vi "AMC100 UI DLL.vi"() -> ()   [LabVIEW 2015]
panel:
  in  "stop":bool
  in  "deviceHandle":i32
  in  "Tab Control":enum32{"Navigation", "Interface", "About"}(tab)
  out "move out":bool caption="Move"
  in  "Positioner 2":u16(ring)=15 caption="Positioner" items=["ECGp5050", "ECGt5050", "ECR3030", "ECR4040", "ECR5050", "ECSx3030", "ECSx3040", "ECSx3050", "ECSx3060", "ECSx3070", "ECSx3080", "ECSx5050", "ECSxy5050", "ECSz3030", "ECSz5050", "EOP1", "EOP2"]
  out "in target range3":bool
  in  "Target Range 3":u32 caption="Target Range"
  in  "Reset Error 2":bool
  in  "Reset Error 3":bool
  out "Error 3":bool caption="Error"
  out "Error Message 3":string
  out "actor type 3":u16(ring) caption="Status" items=["linear positioner"=0, "goniometer"=1, "rotator"=2, "< error >"=9]
  out "actor type 2":u16(ring) caption="Status" items=["linear positioner"=0, "rotator"=1, "goniometer"=2, "< error >"=9]
  out "actor type":u16(ring) caption="Status" items=["linear positioner"=0, "rotator"=1, "goniometer"=2, "< error >"=9]
  out "EotLeftDetected3":bool caption="Status Eot BWD"
  out "EotrightDetected3":bool caption="Status Eot FWD"
  in  "EoT 3":bool=TRUE caption="Stop on EoT"
  out "EotLeftDetected2":bool caption="Status Eot BWD"
  out "EotrightDetected2":bool caption="Status Eot FWD"
  in  "EoT 2":bool=TRUE caption="Stop on EoT"
  in  "Move 3":bool
  out "MoveSignal 3":bool caption="Move"
  out "MoveSignal":bool caption="Move"
  out "ReferenceSignal":bool=TRUE
  in  "Axis 3":bool caption="Closed Loop Funktions"
  in  "Axis 2":bool caption="Closed Loop Funktions"
  in  "Target Position 3":i32 caption="Target Position [µm]"
  in  "Target Position 1":i32 caption="Target position [µm]"
  in  "Number of steps 3":i32=1 caption="Number of Steps"
  in  "Number of steps 2":i32=1 caption="Number of Steps"
  in  "Output 2":bool caption="Axis 2"
  in  "Move 2":bool
  in  "Move":bool
  out "ReferenceSignal 3":bool
  out "Reference 3":dbl caption="Reference position [µm]" format="%#_6f"
  in  "Output":bool=TRUE caption="Axis 1"
  out "Output Status 3":bool caption="Output Status"
  out "Error Message":string
  out "Error":bool
  in  "Output 3":bool caption="Axis 3"
  out "Output Status 1":bool=TRUE caption="Output Status"
  out "Position 3":dbl caption="Position [µm]" format="%#_10g"
  out "Output Status 2":bool caption="Output Status"
  in  "auto Reset 3":bool=TRUE caption="Auto Reset"
  in  "amplitude [V] 3":dbl=45.001 caption="Amplitude [V]" format="%#.3f"
  in  "frequency [Hz] 3":dbl=997.363 caption="Frequency [Hz]" format="%#.3f"
  out "Error 2":bool caption="Error"
  out "Error Message 2":string
  out "Connected 3":bool caption="Positioner Connected/Moving"
  in  "Single Step Left 3":bool caption="Open Loop Funktions"
  in  "Positioner 3":u16(ring)=15 caption="Positioner" items=["ECGp5050", "ECGt5050", "ECR3030", "ECR4040", "ECR5050", "ECSx3030", "ECSx3040", "ECSx3050", "ECSx3060", "ECSx3070", "ECSx3080", "ECSx5050", "ECSxy5050", "ECSz3030", "ECSz5050", "EOP1", "EOP2"]
  in  "Endless Left 3":bool caption="Continuous Backward"
  in  "Continuous Forward":bool
  in  "Single Step Right 3":bool caption="Step(s)"
  in  "Fixed DC 3":i32 caption="DC Level"
  out "move out 3":bool caption="Move"
  out "Position 2":i32 caption="Position [µm]"
  in  "amplitude [V] 2":dbl=45.001 caption="Amplitude [V]" format="%#.3f"
  in  "Reference Auto Update 3":bool=TRUE caption="Auto Update"
  in  "Amplitude [V]":dbl=45.001 format="%#.3f"
  in  "frequency [Hz] 2":dbl=997.363 caption="Frequency [Hz]" format="%#.3f"
  in  "Reference Auto Update 1":bool=TRUE caption="Auto Update"
  in  "Frequency [Hz]":dbl=1998.531 format="%#.3f"
  out "Connected 2":bool caption="Positioner Connected/Moving"
  in  "Single Step Left":bool caption="Open Loop Funktions"
  in  "Single Step Left 2":bool caption="Open Loop Funktions"
  in  "Single Step Right 2":bool caption="Step(s)"
  in  "Number of steps 1":i32=1 caption="Number of Steps"
  out "ReferenceSignal 2":bool
  in  "Single Step Right":bool caption="Step(s)"
  in  "Endless Left":bool caption="Continuous Backward"
  in  "Continuous Forward":bool
  in  "Endless Left 2":bool caption="Continuous Backward"
  out "EotLeftDetected1":bool caption="Status Eot BWD"
  out "EotrightDetected1":bool caption="Status Eot FWD"
  in  "EoT 1":bool caption="Stop on EoT"
  in  "Target position 2":i32 caption="Target Position [µm]"
  out "in target range2":bool
  in  "Continuous Forward":bool
  out "Reference 2":i32 caption="Reference position [µm]"
  in  "Fixed DC 2":i32 caption="DC Level"
  out "MoveSignal 2":bool caption="Move"
  out "in target range1":bool
  in  "Target Range 2":u32 caption="Target Range"
  in  "Target Range 1":u32 caption="Target Range"
  out "Reference":dbl=-7597148.0 caption="Reference position [µm]" format="%#_6f"
  out "Position":dbl=14701.126 caption="Position [µm]" format="%#_10f"
  in  "Axis 1":bool caption="Closed Loop Funktions"
  in  "auto Reset 1":bool=TRUE caption="Auto Reset"
  in  "Fixed DC 1":i32 caption="DC Level"
  out "move out 2":bool caption="Move"
  in  "auto Reset 2":bool=TRUE caption="Auto Reset"
  in  "Reference Auto Update 2":bool=TRUE caption="Auto Update"
  in  "Reset Error":bool
  in  "Axes halt":bool=TRUE
  out "Connected":bool=TRUE caption="Positioner Connected/Moving"
  in  "Positioner":u16(ring)=15 items=["ECGp5050", "ECGt5050", "ECR3030", "ECR4040", "ECR5050", "ECSx3030", "ECSx3040", "ECSx3050", "ECSx3060", "ECSx3070", "ECSx3080", "ECSx5050", "ECSxy5050", "ECSz3030", "ECSz5050", "EOP1", "EOP2"]
  in  "RT in move 3":bool=TRUE caption="Move"
  in  "Steps per pulse 3":i32 caption="Steps per pulse [Steps]"
  out "RT in move Signal 3":bool=TRUE caption="move"
  in  "Mode Input 3":u16(ring) caption="Mode" items=["Trigger (LVDS)"=11, "Trigger (LVTTL)"=10, "Stepper (LVDS)"=9, "Stepper (LVTTL)"=8, "AquadB (LVDS)"=1, "AquadB (LVTTL)"=0, "OFF"=15]
  in  "Loop Mode 3":u16(ring) caption="Loop mode" items=["closed-loop"=1, "open-loop"=0]
  in  "Change per pulse 3":i32 caption="Change per pulse  [u°/nm]"
  in  "RT in move 2":bool=TRUE caption="Move"
  in  "Steps per pulse 2":i32 caption="Steps per pulse [Steps]"
  out "RT in move Signal 2":bool=TRUE caption="move"
  in  "Mode Input 2":u16(ring) caption="Mode" items=["Trigger (LVDS)"=11, "Trigger (LVTTL)"=10, "Stepper (LVDS)"=9, "Stepper (LVTTL)"=8, "AquadB (LVDS)"=1, "AquadB (LVTTL)"=0, "OFF"=15]
  in  "Loop Mode 2":u16(ring) caption="Loop mode" items=["closed-loop"=1, "open-loop"=0]
  in  "Change per pulse 2":i32 caption="Change per pulse  [u°/nm]"
  in  "Output Mode":u16(ring) caption="Mode" items=["AquadB (LVTTL)", "AquadB (LVDS)"]
  in  "RT in move 1":bool=TRUE caption="Move"
  in  "AquadB Resolution 3":i32 caption="AquadB Resolution [nm]"
  in  "AqaudB clock 2":i32 caption="AquadB Clock [ns]"
  in  "AqaudB clock 1":i32 caption="AquadB Clock [ns]"
  in  "AquadB Resolution 2":i32 caption="AquadB Resolution [nm]"
  in  "AquadB out 1":bool caption="AquadB enable"
  in  "Steps per pulse 1":i32 caption="Steps per pulse [Steps]"
  in  "AquadB out 3":bool caption="AquadB enable"
  in  "AquadB in res 1":i32 caption="AquadB Resolution [nm]"
  in  "AquadB Resolution 1":i32 caption="AquadB Resolution [nm]"
  in  "AquadB out 2":bool caption="AquadB enable"
  in  "AqaudB clock 3":i32 caption="AquadB Clock [ns]"
  in  "Reset Error 6":bool
  in  "Reset Error 5":bool
  out "Error Message 5":string
  out "Error 5":bool caption="Error"
  out "Error Message 6":string
  out "Error 6":bool caption="Error"
  in  "AquadB in res 3":i32 caption="AquadB Resolution [nm]"
  in  "AquadB in res 2":i32 caption="AquadB Resolution [nm]"
  in  "Reset Error 4":bool
  out "RT in move Signal 1":bool=TRUE caption="move"
  in  "Mode Input 1":u16(ring) caption="Mode" items=["Trigger (LVDS)"=11, "Trigger (LVTTL)"=10, "Stepper (LVDS)"=9, "Stepper (LVTTL)"=8, "AquadB (LVDS)"=1, "AquadB (LVTTL)"=0, "OFF"=15]
  out "Error Message 4":string
  out "Error 4":bool caption="Error"
  in  "Loop Mode 1":u16(ring) caption="Loop mode" items=["closed-loop"=1, "open-loop"=0]
  in  "Change per pulse 1":i32 caption="Change per pulse [u°/nm]"
  in  "Reset Error 7":bool
  in  "Factory Reset":bool
  in  "Reboot":bool
  out "Error Message 7":string
  in  "Lock password":string
  in  "name":string="Test" caption="Device Name"
  in  "Access Password":string
  out "locked":bool
  out "authorized":bool
  out "Error 7":bool caption="Error"
  in  "Unlock":bool=TRUE
  out "Name":string caption="Device Name"
  out "Device type":string="AMC100/NUM"
  out "Mac Adress":string="70:B3:D5:D7:61:E1"
  out "Sn":string caption="Serial Number"
  out "ip":string="192.168.1.1" caption="IP Adress"
  out "Firmware":string caption="Firmware Version"
  out "FPGA":string caption="FPGA Version"
  # "Real Time Output"
  # "Real Time Input"
  # "Global Parameters"
  # "Axis 1"
  # "Axis 1"
  # "Axis 2"
  # "Axis 2"
  # "Axis 3"
  # "Axis 3"
  # "Device Info"
  # "Device Access"
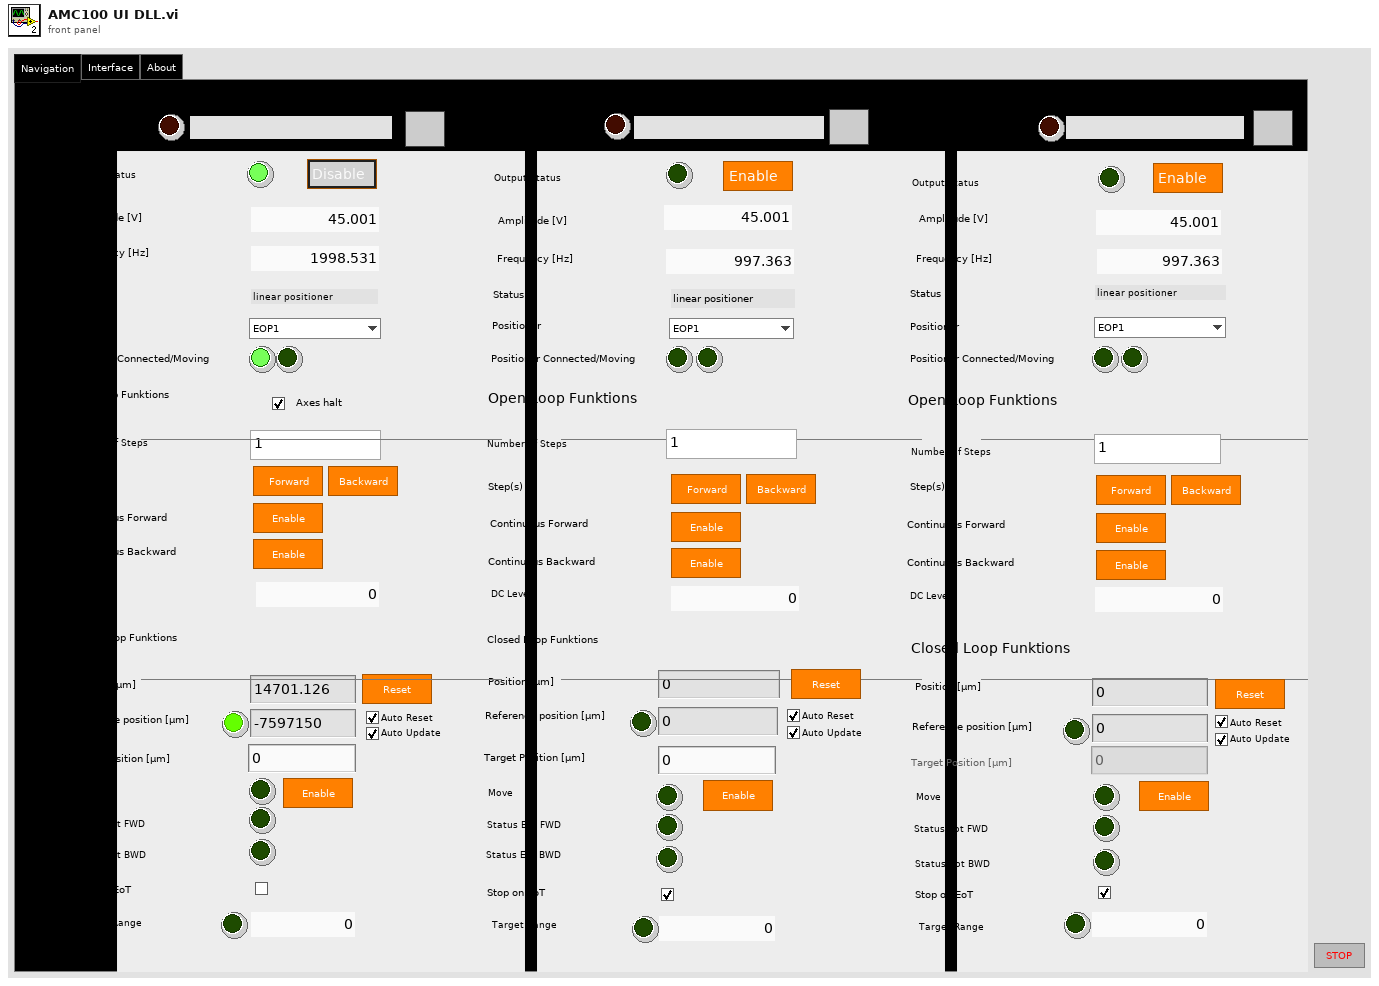
[diagram p1: front panel]
types:
  T1 = enum8{"Enabled", "Disabled", "Disabled and Grayed Out"}
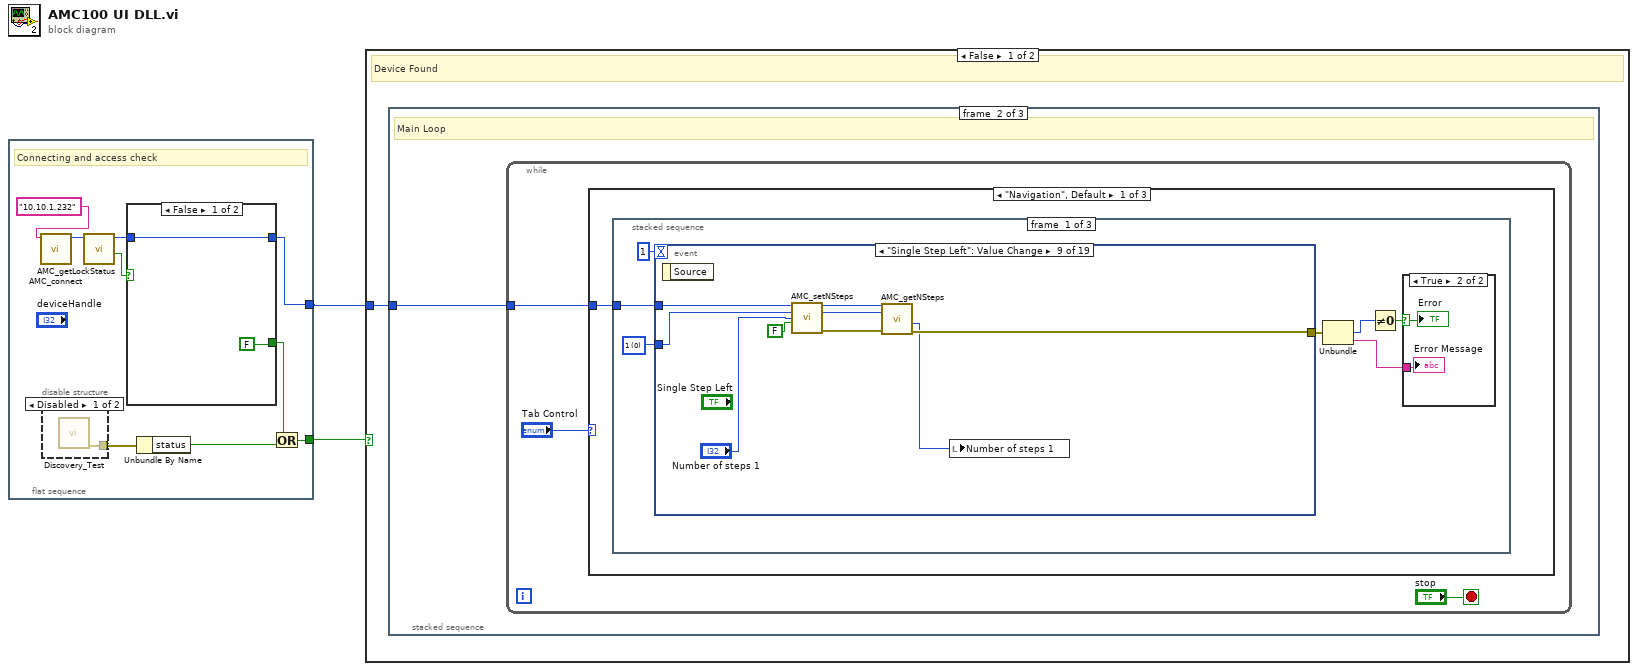
[diagram p0: block diagram]
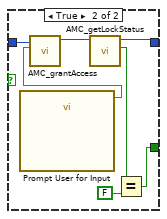
[diagram p3: hidden frame]
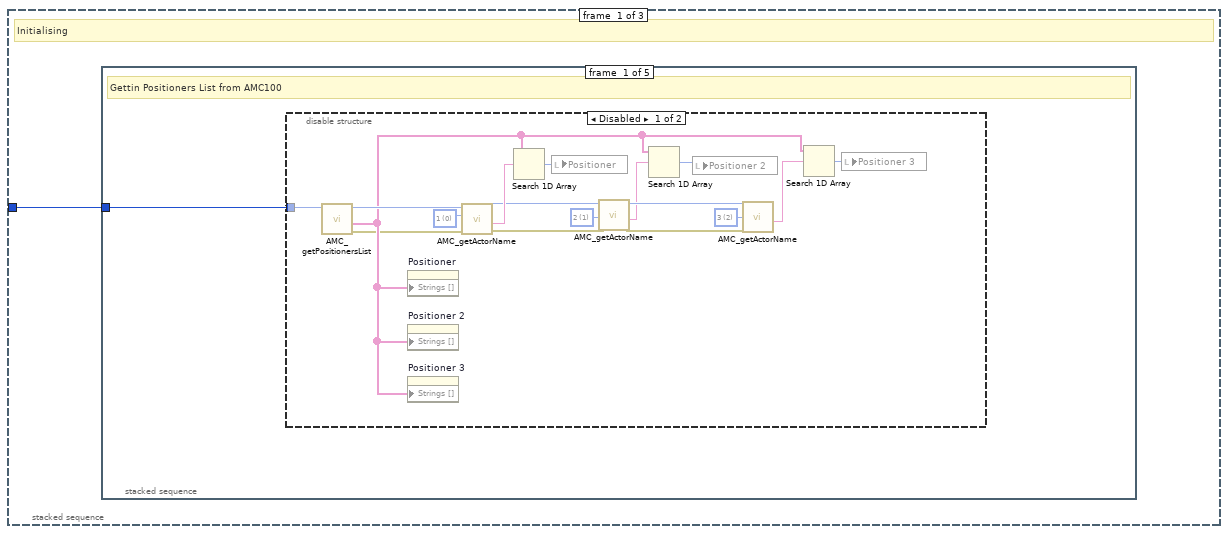
[diagram p4: hidden frame]
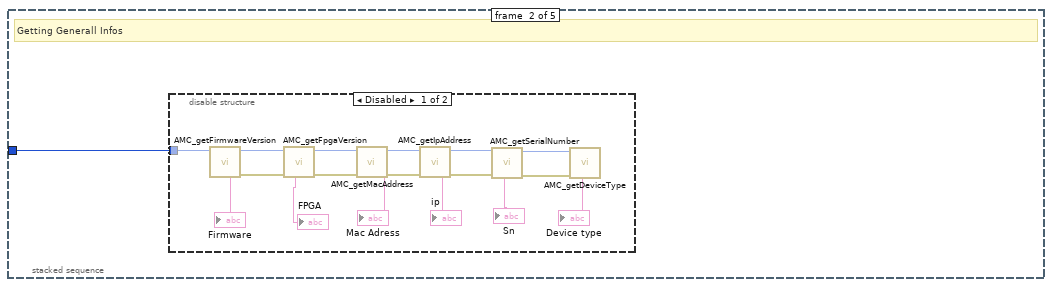
[diagram p6: hidden frame]
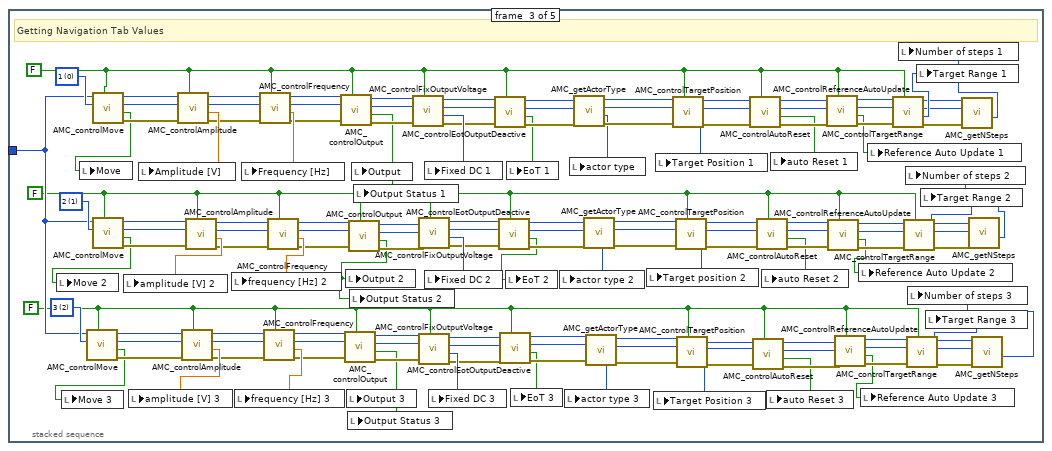
[diagram p8: hidden frame]
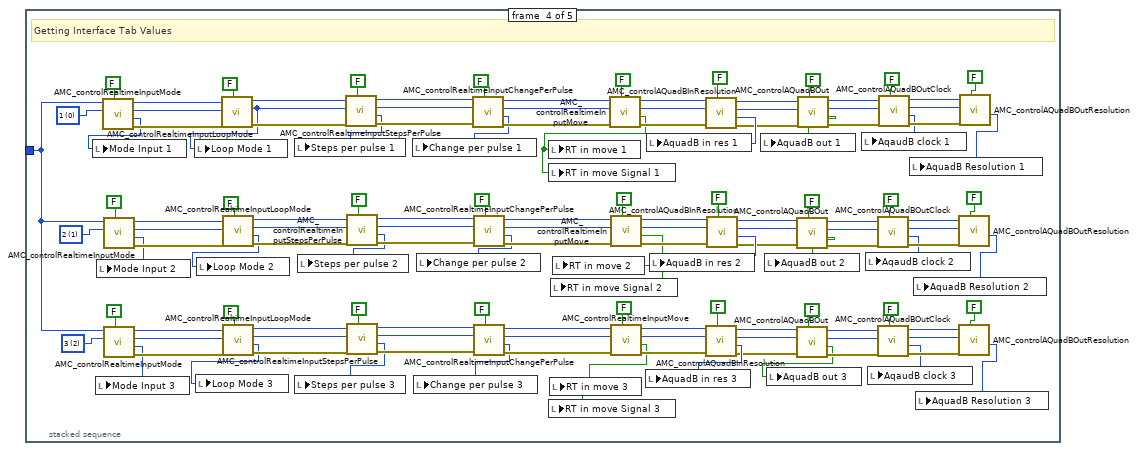
[diagram p9: hidden frame]
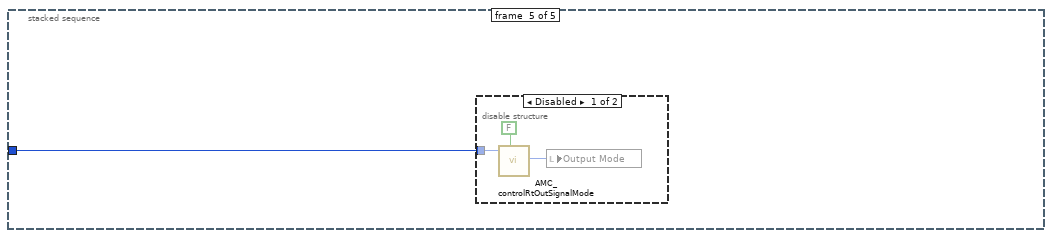
[diagram p10: hidden frame]
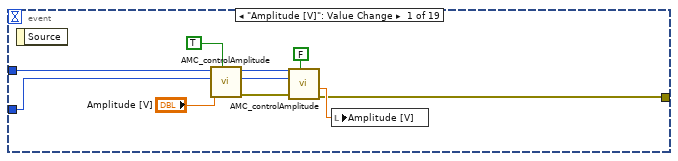
[diagram p13: hidden frame]
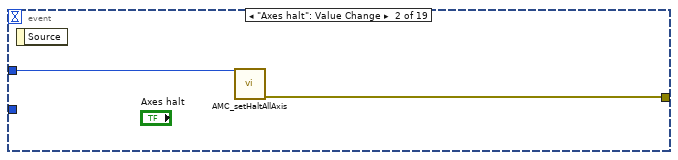
[diagram p14: hidden frame]
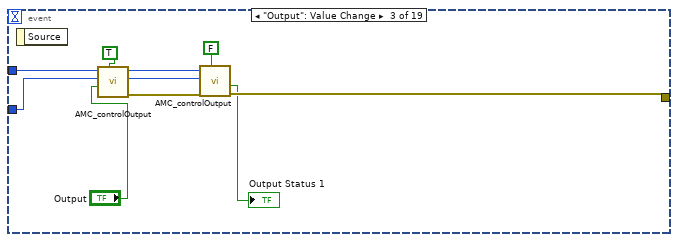
[diagram p15: hidden frame]
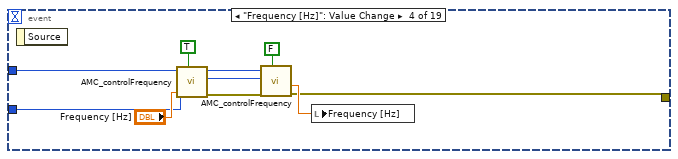
[diagram p16: hidden frame]
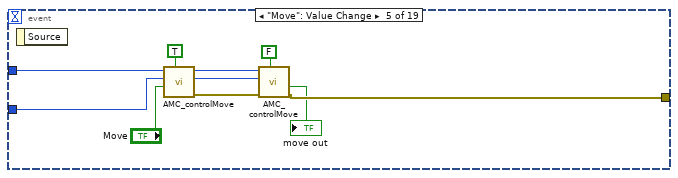
[diagram p17: hidden frame]
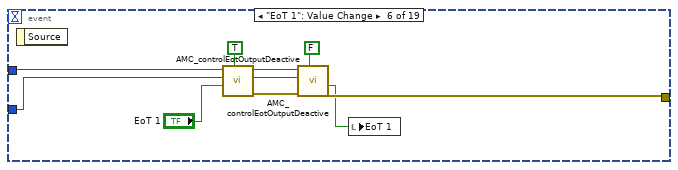
[diagram p18: hidden frame]
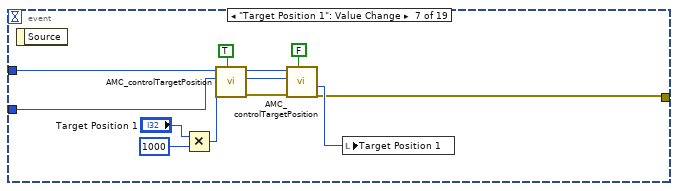
[diagram p19: hidden frame]
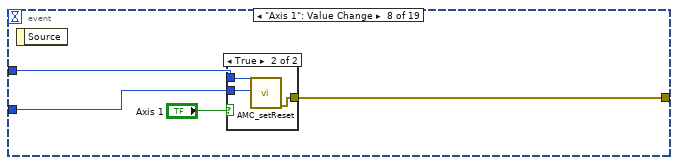
[diagram p20: hidden frame]
diagram:
  n1 = flat-sequence {
    tunnel: [w9] -> w1
    tunnel: [w10] -> w2
    frame #0 {
      # "Connecting and access check"
      n2 = call "AMC_connect.vi"("deviceAddress"="10.10.1.232") -> ("deviceHandle"=w6:i32)  [unwired: 5 in, 1 out]
      n3 = disable-structure shown="Disabled" {
        disable-tunnel: [w12 _] -> w11
        frame Disabled {
          n4 = call "Discovery_Test.vi"() -> ("error out"=w12:errorcluster)  [unwired: 10 in, 1 out]
        }
        frame Enabled {
        }
      }
      n5 = call "AMC_getLockStatus.vi"("deviceHandle"=w6) -> ("locked"=w4:bool, "deviceHandle"=w5:i32)  [unwired: 7 in, 2 out]
      n6 = case shown="False" w4 {
        tunnel: w5 -> [w14 w21]
        tunnel: [w14 w18] -> w10
        tunnel: [FALSE w15] -> w8
        frame False {
        }
        frame True {
          n7 = call "Prompt User for Input"() -> ("password"=w20:string)  [unwired: 17 in, 2 out]
          n8 = call "AMC_grantAccess.vi"("password"=w20, "deviceHandle"=w21) -> ("deviceHandle"=w19:i32)  [unwired: 8 in, 1 out]
          n9 = call "AMC_getLockStatus.vi"("deviceHandle"=w19) -> ("authorized"=w16:bool, "deviceHandle"=w18:i32)  [unwired: 7 in, 2 out]
          n10 = Equal?(x=w16, y=FALSE) -> (x = y?=w15:bool)
        }
      }
      n11 = Unbundle By Name(w11) -> ("status"=w7:bool)
      n12 = Or(x=w8, y=w7) -> (x .or. y?=w9:bool)
    }
  }
  n13 = case shown="False" w1 {
    tunnel: w2 -> [w22 _]
    frame False {
      # "Device Found"
      n14 = stacked-sequence {
        tunnel: w22 -> [w23 w335 w1339]
        frame #0 {
          # "Initialising"
          n15 = stacked-sequence {
            tunnel: w23 -> [w24 w42 w105 w281 w331]
            frame #0 {
              # "Gettin Positioners List from AMC100"
              n16 = disable-structure shown="Disabled" {
                disable-tunnel: w24 -> [w34 _]
                frame Disabled {
                  w36 = u8 2 items=["1", "2", "3"] ("axis")
                  w35 = u8 1 items=["1", "2", "3"] ("axis")
                  w39 = u8 0 items=["1", "2", "3"] ("axis")
                  n17 = call "AMC_getPositionersList.vi"("deviceHandle"=w34) -> ("error out"=w25:errorcluster, "list"=w28:string[], "deviceHandle"=w29:i32)  [unwired: 7 in, 1 out]
                  n18 = property on="Positioner" class="Ring (strict)"("Strings []"=w28) -> ()  [unwired: 2 in, 2 out]
                  n19 = property on="Positioner 2" class="Ring (strict)"("Strings []"=w28) -> ()  [unwired: 2 in, 2 out]
                  n20 = property on="Positioner 3" class="Ring (strict)"("Strings []"=w28) -> ()  [unwired: 2 in, 2 out]
                  n21 = call "AMC_getActorName.vi"("error in"=w25, "axis"=w39, "deviceHandle"=w29) -> ("error out"=w27:errorcluster, "actor name"=w40:string, "deviceHandle"=w38:i32)  [unwired: 5 in, 1 out]
                  n22 = Search 1D Array(1D array=w28, element=w40) -> (index of element=w41:i32)  [unwired: 1 in]
                  n23 = local write "Positioner"(w41) -> ()
                  n24 = call "AMC_getActorName.vi"("error in"=w27, "axis"=w35, "deviceHandle"=w38) -> ("error out"=w26:errorcluster, "actor name"=w31:string, "deviceHandle"=w37:i32)  [unwired: 5 in, 1 out]
                  n25 = Search 1D Array(1D array=w28, element=w31) -> (index of element=w33:i32)  [unwired: 1 in]
                  n26 = local write "Positioner 2"(w33) -> ()
                  n27 = call "AMC_getActorName.vi"("error in"=w26, "axis"=w36, "deviceHandle"=w37) -> ("actor name"=w30:string)  [unwired: 5 in, 3 out]
                  n28 = Search 1D Array(1D array=w28, element=w30) -> (index of element=w32:i32)  [unwired: 1 in]
                  n29 = local write "Positioner 3"(w32) -> ()
                }
                frame Enabled {
                }
              }
            }
            frame #1 {
              # "Getting Generall Infos"
              n30 = disable-structure shown="Disabled" {
                disable-tunnel: w42 -> [w47 _]
                frame Disabled {
                  n31 = call "AMC_getFirmwareVersion.vi"("deviceHandle"=w47) -> ("error out"=w45:errorcluster, "version"=→"Firmware":string, "deviceHandle"=w46:i32)  [unwired: 8 in]
                  n32 = call "AMC_getFpgaVersion.vi"("error in"=w45, "device Handle"=w46) -> ("error out"=w55:errorcluster, "version"=→"FPGA":string, "device Handle"=w59:i32)  [unwired: 7 in]
                  n33 = call "AMC_getMacAddress.vi"("error in"=w55, "deviceHandle"=w59) -> ("error out"=w54:errorcluster, "mac"=→"Mac Adress":string, "deviceHandle"=w57:i32)  [unwired: 7 in]
                  n34 = call "AMC_getIpAddress.vi"("error in"=w54, "device Handle"=w57) -> ("error out"=w51:errorcluster, "ip"=→"ip":string, "device Handle"=w52:i32)  [unwired: 7 in]
                  n35 = call "AMC_getSerialNumber.vi"("error in"=w51, "device Handle"=w52) -> ("error out"=w48:errorcluster, "sn"=→"Sn":string, "device Handle"=w49:i32)  [unwired: 7 in]
                  n36 = call "AMC_getDeviceType.vi"("error in"=w48, "device Handle"=w49) -> ("type"=→"Device type":string)  [unwired: 7 in, 2 out]
                }
                frame Enabled {
                }
              }
            }
            frame #2 {
              w106 = u8 2 items=["1", "2", "3"] ("axis")
              w93 = FALSE ("set")
              w107 = u8 1 items=["1", "2", "3"] ("axis")
              w94 = FALSE ("set")
              w108 = u8 0 items=["1", "2", "3"] ("axis")
              w95 = FALSE ("set")
              # "Getting Navigation Tab Values"
              n37 = call "AMC_controlMove.vi"("set"=w93, "axis"=w106, "deviceHandle"=w105) -> ("error out"=w109:errorcluster, "enable out"=w76:bool, "axis"=w110:u8, "deviceHandle"=w111:i32)  [unwired: 5 in]
              n38 = local write "Move 3"(w76) -> ()
              n39 = call "AMC_controlMove.vi"("set"=w95, "axis"=w108, "deviceHandle"=w105) -> ("error out"=w117:errorcluster, "enable out"=w86:bool, "axis"=w115:u8, "deviceHandle"=w116:i32)  [unwired: 5 in]
              n40 = local write "Move"(w86) -> ()
              n41 = call "AMC_controlMove.vi"("set"=w94, "axis"=w107, "deviceHandle"=w105) -> ("error out"=w112:errorcluster, "enable out"=w81:bool, "axis"=w113:u8, "deviceHandle"=w114:i32)  [unwired: 5 in]
              n42 = local write "Move 2"(w81) -> ()
              n43 = call "AMC_controlAmplitude.vi"("set"=w95, "error in"=w117, "axis"=w115, "deviceHandle"=w116) -> ("error out"=w174:errorcluster, "amplitude [V] out"=w200:dbl, "axis"=w186:u8, "deviceHandle"=w201:i32)  [unwired: 2 in]
              n44 = local write "Amplitude [V]"(w200) -> ()
              n45 = call "AMC_controlAmplitude.vi"("set"=w93, "error in"=w109, "axis"=w110, "deviceHandle"=w111) -> ("error out"=w168:errorcluster, "amplitude [V] out"=w191:dbl, "axis"=w180:u8, "deviceHandle"=w195:i32)  [unwired: 2 in]
              n46 = local write "amplitude [V] 3"(w191) -> ()
              n47 = call "AMC_controlAmplitude.vi"("set"=w94, "error in"=w112, "axis"=w113, "deviceHandle"=w114) -> ("error out"=w171:errorcluster, "amplitude [V] out"=w193:dbl, "axis"=w183:u8, "deviceHandle"=w197:i32)  [unwired: 2 in]
              n48 = local write "amplitude [V] 2"(w193) -> ()
              n49 = call "AMC_controlFrequency.vi"("set"=w95, "error in"=w174, "axis"=w186, "deviceHandle"=w201) -> ("error out"=w173:errorcluster, "frequency [Hz] out"=w199:dbl, "axis"=w185:u8, "deviceHandle"=w198:i32)  [unwired: 4 in]
              n50 = local write "Frequency [Hz]"(w199) -> ()
              n51 = call "AMC_controlFrequency.vi"("set"=w93, "error in"=w168, "axis"=w180, "deviceHandle"=w195) -> ("error out"=w167:errorcluster, "frequency [Hz] out"=w190:dbl, "axis"=w179:u8, "deviceHandle"=w194:i32)  [unwired: 4 in]
              n52 = local write "frequency [Hz] 3"(w190) -> ()
              n53 = call "AMC_controlFrequency.vi"("set"=w94, "error in"=w171, "axis"=w183, "deviceHandle"=w197) -> ("error out"=w170:errorcluster, "frequency [Hz] out"=w192:dbl, "axis"=w182:u8, "deviceHandle"=w196:i32)  [unwired: 4 in]
              n54 = local write "frequency [Hz] 2"(w192) -> ()
              n55 = call "AMC_controlOutput.vi"("set"=w95, "error in"=w173, "axis"=w185, "deviceHandle"=w198) -> ("error out"=w172:errorcluster, "enable out"=w85:bool, "axis"=w184:u8, "deviceHandle"=w189:i32)  [unwired: 4 in]
              n56 = call "AMC_controlOutput.vi"("set"=w93, "error in"=w167, "axis"=w179, "deviceHandle"=w194) -> ("error out"=w166:errorcluster, "enable out"=w75:bool, "axis"=w178:u8, "deviceHandle"=w187:i32)  [unwired: 4 in]
              n57 = local write "Output 3"(w75) -> ()
              n58 = local write "Output Status 3"(w75) -> ()
              n59 = call "AMC_controlOutput.vi"("set"=w94, "error in"=w170, "axis"=w182, "deviceHandle"=w196) -> ("error out"=w169:errorcluster, "enable out"=w80:bool, "axis"=w181:u8, "deviceHandle"=w188:i32)  [unwired: 4 in]
              n60 = local write "Output 2"(w80) -> ()
              n61 = local write "Output Status 2"(w80) -> ()
              n62 = local write "Output"(w85) -> ()
              n63 = local write "Output Status 1"(w85) -> ()
              n64 = call "AMC_controlFixOutputVoltage.vi"("set"=w95, "error in"=w172, "axis"=w184, "deviceHandle"=w189) -> ("error out"=w163:errorcluster, "voltage"=w177:i32, "axis"=w164:u8, "deviceHandle"=w165:i32)  [unwired: 4 in]
              n65 = call "AMC_controlFixOutputVoltage.vi"("set"=w94, "error in"=w169, "axis"=w181, "deviceHandle"=w188) -> ("error out"=w160:errorcluster, "voltage"=w176:i32, "axis"=w161:u8, "deviceHandle"=w162:i32)  [unwired: 4 in]
              n66 = call "AMC_controlFixOutputVoltage.vi"("set"=w93, "error in"=w166, "axis"=w178, "deviceHandle"=w187) -> ("error out"=w157:errorcluster, "voltage"=w175:i32, "axis"=w158:u8, "deviceHandle"=w159:i32)  [unwired: 4 in]
              n67 = local write "Fixed DC 1"(w177) -> ()
              n68 = local write "Fixed DC 2"(w176) -> ()
              n69 = local write "Fixed DC 3"(w175) -> ()
              n70 = call "AMC_controlEotOutputDeactive.vi"("set"=w95, "error in"=w163, "axis"=w164, "deviceHandle"=w165) -> ("error out"=w154:errorcluster, "enable out"=w84:bool, "axis"=w155:u8, "deviceHandle"=w156:i32)  [unwired: 4 in]
              n71 = call "AMC_controlEotOutputDeactive.vi"("set"=w94, "error in"=w160, "axis"=w161, "deviceHandle"=w162) -> ("error out"=w151:errorcluster, "enable out"=w79:bool, "axis"=w152:u8, "deviceHandle"=w153:i32)  [unwired: 4 in]
              n72 = call "AMC_controlEotOutputDeactive.vi"("set"=w93, "error in"=w157, "axis"=w158, "deviceHandle"=w159) -> ("error out"=w148:errorcluster, "enable out"=w74:bool, "axis"=w149:u8, "deviceHandle"=w150:i32)  [unwired: 4 in]
              n73 = local write "EoT 2"(w79) -> ()
              n74 = local write "EoT 1"(w84) -> ()
              n75 = local write "EoT 3"(w74) -> ()
              n76 = call "AMC_getActorType.vi"("error in"=w154, "axis"=w155, "deviceHandle"=w156) -> ("error out"=w142:errorcluster, "positioner type"=w89:u16, "axis"=w143:i32, "deviceHandle"=w144:i32)  [unwired: 5 in]
              n77 = local write "actor type"(w89) -> ()
              n78 = call "AMC_getActorType.vi"("error in"=w151, "axis"=w152, "deviceHandle"=w153) -> ("error out"=w145:errorcluster, "positioner type"=w88:u16, "axis"=w146:i32, "deviceHandle"=w147:i32)  [unwired: 5 in]
              n79 = local write "actor type 2"(w88) -> ()
              n80 = call "AMC_getActorType.vi"("error in"=w148, "axis"=w149, "deviceHandle"=w150) -> ("error out"=w139:errorcluster, "positioner type"=w87:u16, "axis"=w140:i32, "deviceHandle"=w141:i32)  [unwired: 5 in]
              n81 = local write "actor type 3"(w87) -> ()
              n82 = call "AMC_controlTargetPosition.vi"("set"=w95, "error in"=w142, "axis"=w143, "deviceHandle"=w144) -> ("error out"=w135:errorcluster, "target out"=w138:i32, "axis"=w131:u8, "deviceHandle"=w133:i32)  [unwired: 4 in]
              n83 = local write "Target Position 1"(w138) -> ()
              n84 = call "AMC_controlTargetPosition.vi"("set"=w94, "error in"=w145, "axis"=w146, "deviceHandle"=w147) -> ("error out"=w129:errorcluster, "target out"=w137:i32, "axis"=w125:u8, "deviceHandle"=w127:i32)  [unwired: 4 in]
              n85 = local write "Target position 2"(w137) -> ()
              n86 = call "AMC_controlTargetPosition.vi"("set"=w93, "error in"=w139, "axis"=w140, "deviceHandle"=w141) -> ("error out"=w123:errorcluster, "target out"=w136:i32, "axis"=w119:u8, "deviceHandle"=w121:i32)  [unwired: 4 in]
              n87 = local write "Target Position 3"(w136) -> ()
              n88 = call "AMC_controlAutoReset.vi"("set"=w95, "error in"=w135, "axis"=w131, "deviceHandle in"=w133) -> ("error out"=w134:errorcluster, "enable out"=w83:bool, "axis"=w130:u8, "deviceHandle out"=w132:i32)  [unwired: 4 in]
              n89 = call "AMC_controlAutoReset.vi"("set"=w93, "error in"=w123, "axis"=w119, "deviceHandle in"=w121) -> ("error out"=w122:errorcluster, "enable out"=w73:bool, "axis"=w118:u8, "deviceHandle out"=w120:i32)  [unwired: 4 in]
              n90 = call "AMC_controlAutoReset.vi"("set"=w94, "error in"=w129, "axis"=w125, "deviceHandle in"=w127) -> ("error out"=w128:errorcluster, "enable out"=w78:bool, "axis"=w124:u8, "deviceHandle out"=w126:i32)  [unwired: 4 in]
              n91 = local write "auto Reset 2"(w78) -> ()
              n92 = local write "auto Reset 3"(w73) -> ()
              n93 = local write "auto Reset 1"(w83) -> ()
              n94 = call "AMC_controlReferenceAutoUpdate.vi"("set"=w95, "error in"=w134, "axis"=w130, "deviceHandle"=w132) -> ("error out"=w102:errorcluster, "enable out"=w82:bool, "axis"=w103:u8, "deviceHandle"=w104:i32)  [unwired: 4 in]
              n95 = call "AMC_controlReferenceAutoUpdate.vi"("set"=w94, "error in"=w128, "axis"=w124, "deviceHandle"=w126) -> ("error out"=w99:errorcluster, "enable out"=w77:bool, "axis"=w100:u8, "deviceHandle"=w101:i32)  [unwired: 4 in]
              n96 = call "AMC_controlReferenceAutoUpdate.vi"("set"=w93, "error in"=w122, "axis"=w118, "deviceHandle"=w120) -> ("error out"=w96:errorcluster, "enable out"=w72:bool, "axis"=w97:u8, "deviceHandle"=w98:i32)  [unwired: 4 in]
              n97 = local write "Reference Auto Update 2"(w77) -> ()
              n98 = local write "Reference Auto Update 3"(w72) -> ()
              n99 = local write "Reference Auto Update 1"(w82) -> ()
              n100 = call "AMC_controlTargetRange.vi"("set"=w95, "error in"=w102, "axis"=w103, "deviceHandle"=w104) -> ("error out"=w69:errorcluster, "range out"=w92:u32, "axis"=w70:u8, "deviceHandle"=w71:i32)  [unwired: 4 in]
              n101 = call "AMC_controlTargetRange.vi"("set"=w94, "error in"=w99, "axis"=w100, "deviceHandle"=w101) -> ("error out"=w61:errorcluster, "range out"=w91:u32, "axis"=w67:u8, "deviceHandle"=w68:i32)  [unwired: 4 in]
              n102 = call "AMC_controlTargetRange.vi"("set"=w93, "error in"=w96, "axis"=w97, "deviceHandle"=w98) -> ("error out"=w60:errorcluster, "range out"=w90:u32, "axis"=w65:u8, "deviceHandle"=w66:i32)  [unwired: 4 in]
              n103 = local write "Target Range 1"(w92) -> ()
              n104 = local write "Target Range 2"(w91) -> ()
              n105 = local write "Target Range 3"(w90) -> ()
              n106 = call "AMC_getNSteps.vi"("error in"=w69, "axis"=w70, "deviceHandle"=w71) -> ("n out"=w63:i32)  [unwired: 5 in, 3 out]
              n107 = local write "Number of steps 1"(w63) -> ()
              n108 = call "AMC_getNSteps.vi"("error in"=w61, "axis"=w67, "deviceHandle"=w68) -> ("n out"=w64:i32)  [unwired: 5 in, 3 out]
              n109 = local write "Number of steps 2"(w64) -> ()
              n110 = call "AMC_getNSteps.vi"("error in"=w60, "axis"=w65, "deviceHandle"=w66) -> ("n out"=w62:i32)  [unwired: 5 in, 3 out]
              n111 = local write "Number of steps 3"(w62) -> ()
            }
            frame #3 {
              w279 = u8 2 items=["1", "2", "3"] ("axis")
              w280 = u8 1 items=["1", "2", "3"] ("axis")
              w314 = u8 0 items=["1", "2", "3"] ("axis")
              # "Getting Interface Tab Values"
              n112 = call "AMC_controlRealtimeInputMode.vi"("set"=FALSE, "axis"=w314, "deviceHandle"=w281) -> ("error out"=w319:errorcluster, "mode out"=w264:i32, "axis"=w278:u8, "deviceHandle"=w324:i32)  [unwired: 5 in]
              n113 = local write "Mode Input 1"(w264) -> ()
              n114 = call "AMC_controlRealtimeInputMode.vi"("set"=FALSE, "axis"=w280, "deviceHandle"=w281) -> ("error out"=w309:errorcluster, "mode out"=w258:i32, "axis"=w274:u8, "deviceHandle"=w304:i32)  [unwired: 5 in]
              n115 = local write "Mode Input 2"(w258) -> ()
              n116 = call "AMC_controlRealtimeInputMode.vi"("set"=FALSE, "axis"=w279, "deviceHandle"=w281) -> ("error out"=w286:errorcluster, "mode out"=w252:i32, "axis"=w269:u8, "deviceHandle"=w291:i32)  [unwired: 5 in]
              n117 = local write "Mode Input 3"(w252) -> ()
              n118 = call "AMC_controlRealtimeInputLoopMode.vi"("set"=FALSE, "error in"=w319, "axis"=w278, "deviceHandle"=w324) -> ("error out"=w318:errorcluster, "axis"=w263:u8, "deviceHandle"=w323:i32)  [unwired: 4 in, 1 out]
              n119 = local write "Loop Mode 1"(w263) -> ()
              n120 = call "AMC_controlRealtimeInputLoopMode.vi"("set"=FALSE, "error in"=w309, "axis"=w274, "deviceHandle"=w304) -> ("error out"=w310:errorcluster, "mode out"=w257:i32, "axis"=w273:u8, "deviceHandle"=w305:i32)  [unwired: 4 in]
              n121 = local write "Loop Mode 2"(w257) -> ()
              n122 = call "AMC_controlRealtimeInputLoopMode.vi"("set"=FALSE, "error in"=w286, "axis"=w269, "deviceHandle"=w291) -> ("error out"=w285:errorcluster, "mode out"=w251:i32, "axis"=w268:u8, "deviceHandle"=w290:i32)  [unwired: 4 in]
              n123 = local write "Loop Mode 3"(w251) -> ()
              n124 = call "AMC_controlRealtimeInputStepsPerPulse.vi"("set"=FALSE, "error in"=w318, "axis"=w263, "deviceHandle"=w323) -> ("error out"=w317:errorcluster, "steps out"=w262:i32, "axis"=w277:u8, "deviceHandle"=w322:i32)  [unwired: 4 in]
              n125 = local write "Steps per pulse 1"(w262) -> ()
              n126 = call "AMC_controlRealtimeInputStepsPerPulse.vi"("set"=FALSE, "error in"=w310, "axis"=w273, "deviceHandle"=w305) -> ("error out"=w311:errorcluster, "steps out"=w256:i32, "axis"=w272:u8, "deviceHandle"=w306:i32)  [unwired: 4 in]
              n127 = local write "Steps per pulse 2"(w256) -> ()
              n128 = call "AMC_controlRealtimeInputStepsPerPulse.vi"("set"=FALSE, "error in"=w285, "axis"=w268, "deviceHandle"=w290) -> ("error out"=w284:errorcluster, "steps out"=w250:i32, "axis"=w267:u8, "deviceHandle"=w289:i32)  [unwired: 4 in]
              n129 = local write "Steps per pulse 3"(w250) -> ()
              n130 = call "AMC_controlRealtimeInputChangePerPulse.vi"("set"=FALSE, "error in"=w317, "axis"=w277, "deviceHandle"=w322) -> ("error out"=w316:errorcluster, "change out"=w261:i32, "axis"=w276:u8, "deviceHandle"=w321:i32)  [unwired: 4 in]
              n131 = local write "Change per pulse 1"(w261) -> ()
              n132 = call "AMC_controlRealtimeInputChangePerPulse.vi"("set"=FALSE, "error in"=w311, "axis"=w272, "deviceHandle"=w306) -> ("error out"=w312:errorcluster, "change out"=w255:i32, "axis"=w271:u8, "deviceHandle"=w307:i32)  [unwired: 4 in]
              n133 = local write "Change per pulse 2"(w255) -> ()
              n134 = call "AMC_controlRealtimeInputChangePerPulse.vi"("set"=FALSE, "error in"=w284, "axis"=w267, "deviceHandle"=w289) -> ("error out"=w283:errorcluster, "change out"=w249:i32, "axis"=w266:u8, "deviceHandle"=w288:i32)  [unwired: 4 in]
              n135 = local write "Change per pulse 3"(w249) -> ()
              n136 = call "AMC_controlRealtimeInputMove.vi"("set"=FALSE, "error in"=w316, "axis"=w276, "deviceHandle"=w321) -> ("error out"=w315:errorcluster, "enable out"=w260:bool, "axis"=w275:u8, "deviceHandle"=w320:i32)  [unwired: 4 in]
              n137 = local write "RT in move 1"(w260) -> ()
              n138 = local write "RT in move Signal 1"(w260) -> ()
              n139 = call "AMC_controlRealtimeInputMove.vi"("set"=FALSE, "error in"=w312, "axis"=w271, "deviceHandle"=w307) -> ("error out"=w313:errorcluster, "enable out"=w254:bool, "axis"=w270:u8, "deviceHandle"=w308:i32)  [unwired: 4 in]
              n140 = local write "RT in move Signal 2"(w254) -> ()
              n141 = local write "RT in move 2"(w254) -> ()
              n142 = call "AMC_controlRealtimeInputMove.vi"("set"=FALSE, "error in"=w283, "axis"=w266, "deviceHandle"=w288) -> ("error out"=w282:errorcluster, "enable out"=w248:bool, "axis"=w265:u8, "deviceHandle"=w287:i32)  [unwired: 4 in]
              n143 = local write "RT in move Signal 3"(w248) -> ()
              n144 = local write "RT in move 3"(w248) -> ()
              n145 = call "AMC_controlAQuadBInResolution.vi"("set"=FALSE, "error in"=w315, "axis"=w275, "deviceHandle"=w320) -> ("error out"=w244:errorcluster, "resolution out"=w259:i32, "axis"=w245:u8, "deviceHandle"=w246:i32)  [unwired: 4 in]
              n146 = local write "AquadB in res 1"(w259) -> ()
              n147 = call "AMC_controlAQuadBInResolution.vi"("set"=FALSE, "error in"=w282, "axis"=w265, "deviceHandle"=w287) -> ("error out"=w211:errorcluster, "resolution out"=w247:i32, "axis"=w212:u8, "deviceHandle"=w213:i32)  [unwired: 4 in]
              n148 = local write "AquadB in res 3"(w247) -> ()
              n149 = call "AMC_controlAQuadBInResolution.vi"("set"=FALSE, "error in"=w313, "axis"=w270, "deviceHandle"=w308) -> ("error out"=w214:errorcluster, "resolution out"=w253:i32, "axis"=w215:u8, "deviceHandle"=w216:i32)  [unwired: 4 in]
              n150 = local write "AquadB in res 2"(w253) -> ()
              n151 = call "AMC_controlAQuadBOut.vi"("set"=FALSE, "error in"=w214, "axis"=w215, "deviceHandle"=w216) -> ("error out"=w230:errorcluster, "enable out"=w203:bool, "axis"=w228:u8, "deviceHandle"=w226:i32)  [unwired: 4 in]
              n152 = local write "AquadB out 2"(w203) -> ()
              n153 = call "AMC_controlAQuadBOut.vi"("set"=FALSE, "error in"=w211, "axis"=w212, "deviceHandle"=w213) -> ("error out"=w221:errorcluster, "enable out"=w202:bool, "axis"=w223:u8, "deviceHandle"=w225:i32)  [unwired: 4 in]
              n154 = local write "AquadB out 3"(w202) -> ()
              n155 = call "AMC_controlAQuadBOut.vi"("set"=FALSE, "error in"=w244, "axis"=w245, "deviceHandle"=w246) -> ("error out"=w239:errorcluster, "enable out"=w204:bool, "axis"=w241:u8, "deviceHandle"=w243:i32)  [unwired: 4 in]
              n156 = local write "AquadB out 1"(w204) -> ()
              n157 = call "AMC_controlAQuadBOutClock.vi"("set"=FALSE, "error in"=w230, "axis"=w228, "deviceHandle"=w226) -> ("error out"=w231:errorcluster, "clock out"=w209:i32, "axis"=w229:u8, "deviceHandle"=w227:i32)  [unwired: 4 in]
              n158 = local write "AqaudB clock 2"(w209) -> ()
              n159 = call "AMC_controlAQuadBOutClock.vi"("set"=FALSE, "error in"=w221, "axis"=w223, "deviceHandle"=w225) -> ("error out"=w220:errorcluster, "clock out"=w208:i32, "axis"=w222:u8, "deviceHandle"=w224:i32)  [unwired: 4 in]
              n160 = local write "AqaudB clock 3"(w208) -> ()
              n161 = call "AMC_controlAQuadBOutClock.vi"("set"=FALSE, "error in"=w239, "axis"=w241, "deviceHandle"=w243) -> ("error out"=w238:errorcluster, "clock out"=w210:i32, "axis"=w240:u8, "deviceHandle"=w242:i32)  [unwired: 4 in]
              n162 = local write "AqaudB clock 1"(w210) -> ()
              n163 = call "AMC_controlAQuadBOutResolution.vi"("set"=FALSE, "error in"=w231, "axis"=w229, "deviceHandle"=w227) -> ("resolution out"=w206:i32)  [unwired: 4 in, 3 out]
              n164 = local write "AquadB Resolution 2"(w206) -> ()
              n165 = call "AMC_controlAQuadBOutResolution.vi"("set"=FALSE, "error in"=w220, "axis"=w222, "deviceHandle"=w224) -> ("resolution out"=w205:i32)  [unwired: 4 in, 3 out]
              n166 = local write "AquadB Resolution 3"(w205) -> ()
              n167 = call "AMC_controlAQuadBOutResolution.vi"("set"=FALSE, "error in"=w238, "axis"=w240, "deviceHandle"=w242) -> ("resolution out"=w207:i32)  [unwired: 4 in, 3 out]
              n168 = local write "AquadB Resolution 1"(w207) -> ()
            }
            frame #4 {
              n169 = disable-structure shown="Disabled" {
                disable-tunnel: w331 -> [w334 _]
                frame Disabled {
                  n170 = call "AMC_controlRtOutSignalMode.vi"("deviceHandle"=w334, "set"=FALSE) -> ("mode out"=w332:i32)  [unwired: 6 in, 2 out]
                  n171 = local write "Output Mode"(w332) -> ()
                }
                frame Enabled {
                }
              }
            }
          }
        }
        frame #1 {
          # "Main Loop"
          n172 = while {
            tunnel: w335 -> [w338]
            stop <- "stop" stop-if-true
            n173 = case shown="\"Navigation\", Default" "Tab Control" {
              tunnel: w338 -> [w339 w925 w1311]
              frame "Navigation", Default {
                n174 = stacked-sequence {
                  tunnel: w339 -> [w346 w541 w735]
                  frame #0 {
                    w345 = u8 0 items=["1", "2", "3"] ("axis in")
                    n175 = event shown="[8] \"Single Step Left\": Value Change" {
                      selector: _ -> [_ _ _ _ _ _ _ _ _ _ _ _ _ _ _ _ _ _ _]
                      dyn-events: _ -> [_ _ _ _ _ _ _ _ _ _ _ _ _ _ _ _ _ _ _]
                      timeout: 1 -> [_ _ _ _ _ _ _ _ _ _ _ _ _ _ _ _ _ _ _]
                      tunnel: w346 -> [w351 w360 w368 w380 w390 w399 w412 w415 w428 w433 w441 w451 w461 _ w474 w485 w489 w499 w531]
                      tunnel: w345 -> [w350 _ w369 w378 w389 w398 w411 w414 w426 w432 w439 w449 w462 _ w473 w484 w488 w498 w509]
                      tunnel: [w349 w359 w364 w372 w384 w393 w401 w413 w421 w431 w436 w452 w456 _ w468 w478 _ w497 w508] -> w343
                      event "Amplitude [V]": Value Change {
                        n176 = event-data() -> ()  [unwired: 1 in, 1 out]
                        n177 = call "AMC_controlAmplitude.vi"("set"=TRUE, "amplitude [V] in"="Amplitude [V]", "axis"=w350, "deviceHandle"=w351) -> ("error out"=w355:errorcluster, "axis"=w352:u8, "deviceHandle"=w356:i32)  [unwired: 2 in, 1 out]
                        n178 = call "AMC_controlAmplitude.vi"("set"=FALSE, "error in"=w355, "axis"=w352, "deviceHandle"=w356) -> ("error out"=w349:errorcluster, "amplitude [V] out"=w353:dbl)  [unwired: 2 in, 2 out]
                        n179 = local write "Amplitude [V]"(w353) -> ()
                      }
                      event "Axes halt": Value Change {
                        n180 = event-data() -> ()  [unwired: 1 in, 1 out]
                        n181 = call "AMC_setHaltAllAxis.vi"("deviceHandle"=w360) -> ("error out"=w359:errorcluster)  [unwired: 9 in, 1 out]
                      }
                      event "Output": Value Change {
                        n182 = event-data() -> ()  [unwired: 1 in, 1 out]
                        n183 = call "AMC_controlOutput.vi"("set"=TRUE, "enable in"="Output", "axis"=w369, "deviceHandle"=w368) -> ("error out"=w365:errorcluster, "axis"=w366:u8, "deviceHandle"=w367:i32)  [unwired: 4 in, 1 out]
                        n184 = call "AMC_controlOutput.vi"("set"=FALSE, "error in"=w365, "axis"=w366, "deviceHandle"=w367) -> ("error out"=w364:errorcluster, "enable out"=→"Output Status 1":bool)  [unwired: 4 in, 2 out]
                      }
                      event "Frequency [Hz]": Value Change {
                        n185 = event-data() -> ()  [unwired: 1 in, 1 out]
                        n186 = call "AMC_controlFrequency.vi"("set"=TRUE, "frequency [Hz] in"="Frequency [Hz]", "axis"=w378, "deviceHandle"=w380) -> ("error out"=w375:errorcluster, "axis"=w371:u8, "deviceHandle"=w376:i32)  [unwired: 4 in, 1 out]
                        n187 = call "AMC_controlFrequency.vi"("set"=FALSE, "error in"=w375, "axis"=w371, "deviceHandle"=w376) -> ("error out"=w372:errorcluster, "frequency [Hz] out"=w373:dbl)  [unwired: 4 in, 2 out]
                        n188 = local write "Frequency [Hz]"(w373) -> ()
                      }
                      event "Move": Value Change {
                        n189 = event-data() -> ()  [unwired: 1 in, 1 out]
                        n190 = call "AMC_controlMove.vi"("set"=TRUE, "enable in"="Move", "axis"=w389, "deviceHandle"=w390) -> ("error out"=w385:errorcluster, "axis"=w386:u8, "deviceHandle"=w387:i32)  [unwired: 4 in, 1 out]
                        n191 = call "AMC_controlMove.vi"("set"=FALSE, "error in"=w385, "axis"=w386, "deviceHandle"=w387) -> ("error out"=w384:errorcluster, "enable out"=→"move out":bool)  [unwired: 4 in, 2 out]
                      }
                      event "EoT 1": Value Change {
                        n192 = event-data() -> ()  [unwired: 1 in, 1 out]
                        n193 = call "AMC_controlEotOutputDeactive.vi"("set"=TRUE, "enable in"="EoT 1", "axis"=w398, "deviceHandle"=w399) -> ("error out"=w395:errorcluster, "axis"=w396:u8, "deviceHandle"=w397:i32)  [unwired: 4 in, 1 out]
                        n194 = call "AMC_controlEotOutputDeactive.vi"("set"=FALSE, "error in"=w395, "axis"=w396, "deviceHandle"=w397) -> ("error out"=w393:errorcluster, "enable out"=w391:bool)  [unwired: 4 in, 2 out]
                        n195 = local write "EoT 1"(w391) -> ()
                      }
                      event "Target Position 1": Value Change {
                        n196 = event-data() -> ()  [unwired: 1 in, 1 out]
                        n197 = Multiply(x="Target Position 1", y=1000) -> (x*y=w407:i32)
                        n198 = call "AMC_controlTargetPosition.vi"("set"=TRUE, "target in"=w407, "axis"=w411, "deviceHandle"=w412) -> ("error out"=w404:errorcluster, "axis"=w405:u8, "deviceHandle"=w406:i32)  [unwired: 4 in, 1 out]
                        n199 = call "AMC_controlTargetPosition.vi"("set"=FALSE, "error in"=w404, "axis"=w405, "deviceHandle"=w406) -> ("error out"=w401:errorcluster, "target out"=w402:i32)  [unwired: 4 in, 2 out]
                        n200 = local write "Target Position 1"(w402) -> ()
                      }
                      event "Axis 1": Value Change {
                        n201 = event-data() -> ()  [unwired: 1 in, 1 out]
                        n202 = case shown="True" "Axis 1" {
                          tunnel: w415 -> [_ w418]
                          tunnel: w414 -> [_ w419]
                          tunnel: [_ w417] -> w413
                          frame False {
                          }
                          frame True {
                            n203 = call "AMC_setReset.vi"("axis"=w419, "deviceHandle"=w418) -> ("error out"=w417:errorcluster)  [unwired: 7 in, 2 out]
                          }
                        }
                      }
                      event "Single Step Left": Value Change {
                        n204 = event-data() -> ()  [unwired: 1 in, 1 out]
                        n205 = call "AMC_setNSteps.vi"("deviceHandle"=w428, "axis"=w426, "n in"="Number of steps 1", "backwards"=FALSE) -> ("deviceHandle"=w423:i32, "axis"=w422:i32, "error out"=w424:errorcluster)  [unwired: 8 in, 1 out]
                        n206 = call "AMC_getNSteps.vi"("error in"=w424, "axis"=w422, "deviceHandle"=w423) -> ("error out"=w421:errorcluster, "n out"=w420:i32)  [unwired: 5 in, 2 out]
                        n207 = local write "Number of steps 1"(w420) -> ()
                      }
                      event "Single Step Right": Value Change {
                        n208 = event-data() -> ()  [unwired: 1 in, 1 out]
                        n209 = local read "Number of steps 1"() -> (w429:i32)
                        n210 = call "AMC_setNSteps.vi"("deviceHandle"=w433, "axis"=w432, "n in"=w429, "backwards"=TRUE) -> ("error out"=w431:errorcluster)  [unwired: 8 in, 3 out]
                      }
                      event "Endless Left": Value Change {
                        n211 = event-data() -> ()  [unwired: 1 in, 1 out]
                        n212 = call "AMC_controlContinousFwd.vi"("set"=TRUE, "enable in"=FALSE, "axis"=w439, "deviceHandle"=w441) -> ("axis"=w438:u8, "deviceHandle"=w440:i32)  [unwired: 4 in, 2 out]
                        n213 = local write "Continuous Forward"(FALSE) -> ()
                        n214 = call "AMC_controlContinousBkwd.vi"("set"=TRUE, "enable in"="Endless Left", "axis"=w438, "deviceHandle"=w440) -> ("error out"=w436:errorcluster)  [unwired: 4 in, 3 out]
                      }
                      event "Continuous Forward": Value Change {
                        n215 = event-data() -> ()  [unwired: 1 in, 1 out]
                        n216 = call "AMC_controlContinousBkwd.vi"("set"=TRUE, "enable in"=FALSE, "axis"=w449, "deviceHandle"=w451) -> ("error out"=w447:errorcluster, "axis"=w448:u8, "deviceHandle"=w450:i32)  [unwired: 4 in, 1 out]
                        n217 = call "AMC_controlContinousFwd.vi"("set"=TRUE, "error in"=w447, "enable in"="Continuous Forward", "axis"=w448, "deviceHandle"=w450) -> ("error out"=w452:errorcluster)  [unwired: 3 in, 3 out]
                        n218 = local write "Endless Left"(FALSE) -> ()
                      }
                      event "Fixed DC 1": Value Change {
                        n219 = event-data() -> ()  [unwired: 1 in, 1 out]
                        n220 = call "AMC_controlFixOutputVoltage.vi"("set"=TRUE, "voltage"="Fixed DC 1", "axis"=w462, "deviceHandle"=w461) -> ("error out"=w457:errorcluster, "axis"=w459:u8, "deviceHandle"=w460:i32)  [unwired: 4 in, 1 out]
                        n221 = call "AMC_controlFixOutputVoltage.vi"("set"=FALSE, "error in"=w457, "axis"=w459, "deviceHandle"=w460) -> ("error out"=w456:errorcluster, "voltage"=w455:i32)  [unwired: 4 in, 2 out]
                        n222 = local write "Fixed DC 1"(w455) -> ()
                      }
                      event "Reset Error": Value Change {
                        n223 = event-data() -> ()  [unwired: 1 in, 1 out]
                        n224 = local write "Error Message"("" ("Error Message")) -> ()
                        n225 = local write "Error"(FALSE ("Error")) -> ()
                      }
                      event "Positioner": Value Change {
                        n226 = event-data() -> ()  [unwired: 1 in, 1 out]
                        n227 = property on="Positioner" class="Ring (strict)"() -> ("RingText.Text"=w472:string)  [unwired: 2 in, 2 out]
                        n228 = call "AMC_controlActorSelection.vi"("set"=TRUE, "actor in"=w472, "axis"=w473, "deviceHandle"=w474) -> ("error out"=w470:errorcluster, "axis"=w469:u8, "deviceHandle"=w471:i32)  [unwired: 4 in, 1 out]
                        n229 = call "AMC_getActorType.vi"("error in"=w470, "axis"=w469, "deviceHandle"=w471) -> ("error out"=w468:errorcluster, "positioner type"=→"actor type":u16)  [unwired: 5 in, 2 out]
                      }
                      event "Target Range 1": Value Change {
                        n230 = event-data() -> ()  [unwired: 1 in, 1 out]
                        n231 = call "AMC_controlTargetRange.vi"("set"=TRUE, "range in"="Target Range 1", "axis"=w484, "deviceHandle"=w485) -> ("error out"=w479:errorcluster, "axis"=w480:u8, "deviceHandle"=w481:i32)  [unwired: 4 in, 1 out]
                        n232 = call "AMC_controlTargetRange.vi"("set"=FALSE, "error in"=w479, "axis"=w480, "deviceHandle"=w481) -> ("error out"=w478:errorcluster, "range out"=w476:u32)  [unwired: 4 in, 2 out]
                        n233 = local write "Target Range 1"(w476) -> ()
                      }
                      event "auto Reset 1": Value Change {
                        n234 = event-data() -> ()  [unwired: 1 in, 1 out]
                        n235 = call "AMC_controlAutoReset.vi"("set"=TRUE, "enable in"="auto Reset 1", "axis"=w488, "deviceHandle in"=w489) -> ("error out"=w493:errorcluster, "axis"=w492:u8, "deviceHandle out"=w491:i32)  [unwired: 4 in, 1 out]
                        n236 = call "AMC_controlAutoReset.vi"("set"=FALSE, "error in"=w493, "axis"=w492, "deviceHandle in"=w491) -> ("enable out"=w486:bool)  [unwired: 4 in, 3 out]
                        n237 = local write "auto Reset 1"(w486) -> ()
                      }
                      event "Reference Auto Update 3": Value Change {
                        n238 = event-data() -> ()  [unwired: 1 in, 1 out]
                        n239 = call "AMC_controlReferenceAutoUpdate.vi"("set"=TRUE, "enable in"="Reference Auto Update 1", "axis"=w498, "deviceHandle"=w499) -> ("error out"=w501:errorcluster, "axis"=w503:u8, "deviceHandle"=w502:i32)  [unwired: 4 in, 1 out]
                        n240 = call "AMC_controlReferenceAutoUpdate.vi"("set"=FALSE, "error in"=w501, "axis"=w503, "deviceHandle"=w502) -> ("error out"=w497:errorcluster, "enable out"=w495:bool)  [unwired: 4 in, 2 out]
                        n241 = local write "Reference Auto Update 1"(w495) -> ()
                      }
                      event Timeout {
                        n242 = event-data() -> ()  [unwired: 1 in, 1 out]
                        n243 = call "AMC_getPosition.vi"("axis"=w509, "deviceHandle"=w531) -> ("error out"=w530:errorcluster, "position"=→"Position":i32, "axis"=w523:u8, "deviceHandle"=w524:i32)  [unwired: 6 in]
                        n244 = call "AMC_getReferencePosition.vi"("error in"=w530, "axis"=w523, "deviceHandle"=w524) -> ("error out"=w518:errorcluster, "reference"=→"Reference":i32, "axis"=w520:i32, "deviceHandle"=w522:i32)  [unwired: 5 in]
                        n245 = call "AMC_getStatusConnected.vi"("error in"=w518, "axis"=w520, "deviceHandle"=w522) -> ("error out"=w517:errorcluster, "connected"=→"Connected":bool, "axis"=w519:i32, "deviceHandle"=w521:i32)  [unwired: 5 in]
                        n246 = call "AMC_getStatusMoving.vi"("error in"=w517, "axis"=w519, "deviceHandle"=w521) -> ("error out"=w535:errorcluster, "moving"=→"MoveSignal":bool, "axis"=w532:i32, "deviceHandle"=w536:i32)  [unwired: 5 in]
                        n247 = call "AMC_getStatusReference.vi"("error in"=w535, "axis"=w532, "deviceHandle"=w536) -> ("error out"=w510:errorcluster, "reference valid"=→"ReferenceSignal":bool, "axis"=w511:i32, "deviceHandle"=w512:i32)  [unwired: 5 in]
                        n248 = call "AMC_getStatusEotBkwd.vi"("error in"=w510, "axis"=w511, "deviceHandle"=w512) -> ("error out"=w528:errorcluster, "EotDetected"=→"EotLeftDetected1":bool, "axis"=w526:u8, "deviceHandle"=w527:i32)  [unwired: 5 in]
                        n249 = call "AMC_getStatusEotFwd.vi"("error in"=w528, "axis"=w526, "deviceHandle"=w527) -> ("error out"=w513:errorcluster, "EotDetected"=→"EotrightDetected1":bool, "axis"=w514:u8, "deviceHandle"=w515:i32)  [unwired: 5 in]
                        n250 = call "AMC_getStatusTargetRange.vi"("error in"=w513, "axis"=w514, "deviceHandle"=w515) -> ("error out"=w508:errorcluster, "in target range"=→"in target range1":bool)  [unwired: 5 in, 2 out]
                      }
                    }
                    n251 = Unbundle(w343) -> ("code"=w341:i32, "source"=w342:string)  [unwired: 1 out]
                    n252 = Not Equal To 0?(x=w341) -> (x != 0?=w340:bool)
                    n253 = case shown="True" w340 {
                      selector: w340 -> [_ w347]
                      tunnel: w342 -> [_ w348]
                      frame False {
                      }
                      frame True {
                        "Error Message" <- w348
                        "Error" <- w347
                      }
                    }
                  }
                  frame #1 {
                    w543 = u8 1 items=["1", "2", "3"] ("axis in")
                    n254 = event shown="[7] \"Single Step Left 2\": Value Change" {
                      selector: _ -> [_ _ _ _ _ _ _ _ _ _ _ _ _ _ _ _ _ _]
                      dyn-events: _ -> [_ _ _ _ _ _ _ _ _ _ _ _ _ _ _ _ _ _]
                      timeout: 1 -> [_ _ _ _ _ _ _ _ _ _ _ _ _ _ _ _ _ _]
                      tunnel: w541 -> [w555 w565 w575 w585 w594 w607 w611 w623 w628 w635 w647 w657 _ w670 w680 w684 w693 w723]
                      tunnel: w543 -> [w554 w564 w574 w584 w593 w605 w610 w622 w627 w634 w645 w658 _ w669 w679 w683 w692 w722]
                      tunnel: [w549 w558 w569 w579 w588 w598 w608 w615 w626 w637 w648 w653 _ w664 _ _ _ w705] -> w539
                      event "amplitude [V] 2": Value Change {
                        n255 = event-data() -> ()  [unwired: 1 in, 1 out]
                        n256 = call "AMC_controlAmplitude.vi"("set"=TRUE, "amplitude [V] in"="amplitude [V] 2", "axis"=w554, "deviceHandle"=w555) -> ("error out"=w550:errorcluster, "axis"=w546:u8, "deviceHandle"=w551:i32)  [unwired: 2 in, 1 out]
                        n257 = call "AMC_controlAmplitude.vi"("set"=FALSE, "error in"=w550, "axis"=w546, "deviceHandle"=w551) -> ("error out"=w549:errorcluster, "amplitude [V] out"=w547:dbl)  [unwired: 2 in, 2 out]
                        n258 = local write "amplitude [V] 2"(w547) -> ()
                      }
                      event "Output 2": Value Change {
                        n259 = event-data() -> ()  [unwired: 1 in, 1 out]
                        n260 = call "AMC_controlOutput.vi"("set"=TRUE, "enable in"="Output 2", "axis"=w564, "deviceHandle"=w565) -> ("error out"=w560:errorcluster, "axis"=w561:u8, "deviceHandle"=w562:i32)  [unwired: 4 in, 1 out]
                        n261 = call "AMC_controlOutput.vi"("set"=FALSE, "error in"=w560, "axis"=w561, "deviceHandle"=w562) -> ("error out"=w558:errorcluster, "enable out"=→"Output Status 2":bool)  [unwired: 4 in, 2 out]
                      }
                      event "frequency [Hz] 2": Value Change {
                        n262 = event-data() -> ()  [unwired: 1 in, 1 out]
                        n263 = call "AMC_controlFrequency.vi"("set"=TRUE, "frequency [Hz] in"="frequency [Hz] 2", "axis"=w574, "deviceHandle"=w575) -> ("error out"=w570:errorcluster, "axis"=w566:u8, "deviceHandle"=w571:i32)  [unwired: 4 in, 1 out]
                        n264 = call "AMC_controlFrequency.vi"("set"=FALSE, "error in"=w570, "axis"=w566, "deviceHandle"=w571) -> ("error out"=w569:errorcluster, "frequency [Hz] out"=w567:dbl)  [unwired: 4 in, 2 out]
                        n265 = local write "frequency [Hz] 2"(w567) -> ()
                      }
                      event "Move 2": Value Change {
                        n266 = event-data() -> ()  [unwired: 1 in, 1 out]
                        n267 = call "AMC_controlMove.vi"("set"=TRUE, "enable in"="Move 2", "axis"=w584, "deviceHandle"=w585) -> ("error out"=w580:errorcluster, "axis"=w581:u8, "deviceHandle"=w582:i32)  [unwired: 4 in, 1 out]
                        n268 = call "AMC_controlMove.vi"("set"=FALSE, "error in"=w580, "axis"=w581, "deviceHandle"=w582) -> ("error out"=w579:errorcluster, "enable out"=→"move out 2":bool)  [unwired: 4 in, 2 out]
                      }
                      event "EoT 2": Value Change {
                        n269 = event-data() -> ()  [unwired: 1 in, 1 out]
                        n270 = call "AMC_controlEotOutputDeactive.vi"("set"=TRUE, "enable in"="EoT 2", "axis"=w593, "deviceHandle"=w594) -> ("error out"=w590:errorcluster, "axis"=w591:u8, "deviceHandle"=w592:i32)  [unwired: 4 in, 1 out]
                        n271 = call "AMC_controlEotOutputDeactive.vi"("set"=FALSE, "error in"=w590, "axis"=w591, "deviceHandle"=w592) -> ("error out"=w588:errorcluster, "enable out"=w586:bool)  [unwired: 4 in, 2 out]
                        n272 = local write "EoT 2"(w586) -> ()
                      }
                      event "Target position 2": Value Change {
                        n273 = event-data() -> ()  [unwired: 1 in, 1 out]
                        n274 = Multiply(x="Target position 2", y=1000) -> (x*y=w603:i32)
                        n275 = call "AMC_controlTargetPosition.vi"("set"=TRUE, "target in"=w603, "axis"=w605, "deviceHandle"=w607) -> ("error out"=w600:errorcluster, "axis"=w599:u8, "deviceHandle"=w601:i32)  [unwired: 4 in, 1 out]
                        n276 = call "AMC_controlTargetPosition.vi"("set"=FALSE, "error in"=w600, "axis"=w599, "deviceHandle"=w601) -> ("error out"=w598:errorcluster, "target out"=w597:i32)  [unwired: 4 in, 2 out]
                        n277 = local write "Target position 2"(w597) -> ()
                      }
                      event "Axis 2": Value Change {
                        n278 = event-data() -> ()  [unwired: 1 in, 1 out]
                        n279 = case shown="True" "Axis 2" {
                          tunnel: w611 -> [_ w613]
                          tunnel: w610 -> [_ w614]
                          tunnel: [_ w612] -> w608
                          frame False {
                          }
                          frame True {
                            n280 = call "AMC_setReset.vi"("axis"=w614, "deviceHandle"=w613) -> ("error out"=w612:errorcluster)  [unwired: 7 in, 2 out]
                          }
                        }
                      }
                      event "Single Step Left 2": Value Change {
                        n281 = event-data() -> ()  [unwired: 1 in, 1 out]
                        n282 = call "AMC_setNSteps.vi"("deviceHandle"=w623, "axis"=w622, "n in"="Number of steps 2", "backwards"=FALSE) -> ("deviceHandle"=w618:i32, "axis"=w617:i32, "error out"=w619:errorcluster)  [unwired: 8 in, 1 out]
                        n283 = call "AMC_getNSteps.vi"("error in"=w619, "axis"=w617, "deviceHandle"=w618) -> ("error out"=w615:errorcluster, "n out"=w616:i32)  [unwired: 5 in, 2 out]
                        n284 = local write "Number of steps 2"(w616) -> ()
                      }
                      event "Single Step Right 2": Value Change {
                        n285 = event-data() -> ()  [unwired: 1 in, 1 out]
                        n286 = local read "Number of steps 2"() -> (w624:i32)
                        n287 = call "AMC_setNSteps.vi"("deviceHandle"=w628, "axis"=w627, "n in"=w624, "backwards"=TRUE) -> ("error out"=w626:errorcluster)  [unwired: 8 in, 3 out]
                      }
                      event "Endless Left 2": Value Change {
                        n288 = event-data() -> ()  [unwired: 1 in, 1 out]
                        n289 = call "AMC_controlContinousFwd.vi"("set"=TRUE, "enable in"=FALSE, "axis"=w634, "deviceHandle"=w635) -> ("error out"=w632:errorcluster, "axis"=w633:u8, "deviceHandle"=w636:i32)  [unwired: 4 in, 1 out]
                        n290 = call "AMC_controlContinousBkwd.vi"("set"=TRUE, "error in"=w632, "enable in"="Endless Left 2", "axis"=w633, "deviceHandle"=w636) -> ("error out"=w637:errorcluster)  [unwired: 3 in, 3 out]
                        n291 = local write "Continuous Forward"(FALSE) -> ()
                      }
                      event "Continuous Forward": Value Change {
                        n292 = event-data() -> ()  [unwired: 1 in, 1 out]
                        n293 = call "AMC_controlContinousBkwd.vi"("set"=TRUE, "enable in"=FALSE, "axis"=w645, "deviceHandle"=w647) -> ("error out"=w643:errorcluster, "axis"=w644:u8, "deviceHandle"=w646:i32)  [unwired: 4 in, 1 out]
                        n294 = call "AMC_controlContinousFwd.vi"("set"=TRUE, "error in"=w643, "enable in"="Continuous Forward", "axis"=w644, "deviceHandle"=w646) -> ("error out"=w648:errorcluster)  [unwired: 3 in, 3 out]
                        n295 = local write "Endless Left 2"(FALSE ("Endless Left 2")) -> ()
                      }
                      event "Fixed DC 2": Value Change {
                        n296 = event-data() -> ()  [unwired: 1 in, 1 out]
                        n297 = call "AMC_controlFixOutputVoltage.vi"("set"=TRUE, "voltage"="Fixed DC 2", "axis"=w658, "deviceHandle"=w657) -> ("error out"=w654:errorcluster, "axis"=w655:u8, "deviceHandle"=w656:i32)  [unwired: 4 in, 1 out]
                        n298 = call "AMC_controlFixOutputVoltage.vi"("set"=FALSE, "error in"=w654, "axis"=w655, "deviceHandle"=w656) -> ("error out"=w653:errorcluster, "voltage"=w651:i32)  [unwired: 4 in, 2 out]
                        n299 = local write "Fixed DC 2"(w651) -> ()
                      }
                      event "Reset Error 2": Value Change {
                        n300 = event-data() -> ()  [unwired: 1 in, 1 out]
                        n301 = local write "Error Message 2"("" ("Error Message 2")) -> ()
                        n302 = local write "Error 2"(FALSE ("Error 2")) -> ()
                      }
                      event "Positioner 2": Value Change {
                        n303 = event-data() -> ()  [unwired: 1 in, 1 out]
                        n304 = property on="Positioner 2" class="Ring (strict)"() -> ("RingText.Text"=w668:string)  [unwired: 2 in, 2 out]
                        n305 = call "AMC_controlActorSelection.vi"("set"=TRUE, "actor in"=w668, "axis"=w669, "deviceHandle"=w670) -> ("error out"=w665:errorcluster, "axis"=w666:u8, "deviceHandle"=w667:i32)  [unwired: 4 in, 1 out]
                        n306 = call "AMC_getActorType.vi"("error in"=w665, "axis"=w666, "deviceHandle"=w667) -> ("error out"=w664:errorcluster, "positioner type"=→"actor type 2":u16)  [unwired: 5 in, 2 out]
                      }
                      event "Target Range 2": Value Change {
                        n307 = event-data() -> ()  [unwired: 1 in, 1 out]
                        n308 = call "AMC_controlTargetRange.vi"("set"=TRUE, "range in"="Target Range 2", "axis"=w679, "deviceHandle"=w680) -> ("error out"=w674:errorcluster, "axis"=w675:u8, "deviceHandle"=w676:i32)  [unwired: 4 in, 1 out]
                        n309 = call "AMC_controlTargetRange.vi"("set"=FALSE, "error in"=w674, "axis"=w675, "deviceHandle"=w676) -> ("range out"=w672:u32)  [unwired: 4 in, 3 out]
                        n310 = local write "Target Range 2"(w672) -> ()
                      }
                      event "auto Reset 2": Value Change {
                        n311 = event-data() -> ()  [unwired: 1 in, 1 out]
                        n312 = call "AMC_controlAutoReset.vi"("set"=TRUE, "enable in"="auto Reset 2", "axis"=w683, "deviceHandle in"=w684) -> ("error out"=w688:errorcluster, "axis"=w687:u8, "deviceHandle out"=w686:i32)  [unwired: 4 in, 1 out]
                        n313 = call "AMC_controlAutoReset.vi"("set"=FALSE, "error in"=w688, "axis"=w687, "deviceHandle in"=w686) -> ("enable out"=w681:bool)  [unwired: 4 in, 3 out]
                        n314 = local write "auto Reset 2"(w681) -> ()
                      }
                      event "Reference Auto Update 2": Value Change {
                        n315 = event-data() -> ()  [unwired: 1 in, 1 out]
                        n316 = call "AMC_controlReferenceAutoUpdate.vi"("set"=TRUE, "enable in"="Reference Auto Update 2", "axis"=w692, "deviceHandle"=w693) -> ("error out"=w695:errorcluster, "axis"=w697:u8, "deviceHandle"=w696:i32)  [unwired: 4 in, 1 out]
                        n317 = call "AMC_controlReferenceAutoUpdate.vi"("set"=FALSE, "error in"=w695, "axis"=w697, "deviceHandle"=w696) -> ("enable out"=w690:bool)  [unwired: 4 in, 3 out]
                        n318 = local write "Reference Auto Update 2"(w690) -> ()
                      }
                      event Timeout {
                        n319 = event-data() -> ()  [unwired: 1 in, 1 out]
                        n320 = call "AMC_getPosition.vi"("axis"=w722, "deviceHandle"=w723) -> ("error out"=w721:errorcluster, "position"=→"Position 2":i32, "axis"=w727:u8, "deviceHandle"=w728:i32)  [unwired: 6 in]
                        n321 = call "AMC_getReferencePosition.vi"("error in"=w721, "axis"=w727, "deviceHandle"=w728) -> ("error out"=w711:errorcluster, "reference"=→"Reference 2":i32, "axis"=w713:i32, "deviceHandle"=w715:i32)  [unwired: 5 in]
                        n322 = call "AMC_getStatusConnected.vi"("error in"=w711, "axis"=w713, "deviceHandle"=w715) -> ("error out"=w710:errorcluster, "connected"=→"Connected 2":bool, "axis"=w712:i32, "deviceHandle"=w714:i32)  [unwired: 5 in]
                        n323 = call "AMC_getStatusMoving.vi"("error in"=w710, "axis"=w712, "deviceHandle"=w714) -> ("error out"=w729:errorcluster, "moving"=→"MoveSignal 2":bool, "axis"=w724:i32, "deviceHandle"=w730:i32)  [unwired: 5 in]
                        n324 = call "AMC_getStatusReference.vi"("error in"=w729, "axis"=w724, "deviceHandle"=w730) -> ("error out"=w702:errorcluster, "reference valid"=→"ReferenceSignal 2":bool, "axis"=w703:i32, "deviceHandle"=w704:i32)  [unwired: 5 in]
                        n325 = call "AMC_getStatusEotBkwd.vi"("error in"=w702, "axis"=w703, "deviceHandle"=w704) -> ("error out"=w717:errorcluster, "EotDetected"=→"EotLeftDetected2":bool, "axis"=w718:u8, "deviceHandle"=w719:i32)  [unwired: 5 in]
                        n326 = call "AMC_getStatusEotFwd.vi"("error in"=w717, "axis"=w718, "deviceHandle"=w719) -> ("error out"=w706:errorcluster, "EotDetected"=→"EotrightDetected2":bool, "axis"=w707:u8, "deviceHandle"=w708:i32)  [unwired: 5 in]
                        n327 = call "AMC_getStatusTargetRange.vi"("error in"=w706, "axis"=w707, "deviceHandle"=w708) -> ("error out"=w705:errorcluster, "in target range"=→"in target range2":bool)  [unwired: 5 in, 2 out]
                      }
                    }
                    n328 = Unbundle(w539) -> ("code"=w538:i32, "source"=w540:string)  [unwired: 1 out]
                    n329 = Not Equal To 0?(x=w538) -> (x != 0?=w537:bool)
                    n330 = case shown="True" w537 {
                      selector: w537 -> [_ w544]
                      tunnel: w540 -> [_ w545]
                      frame False {
                      }
                      frame True {
                        "Error Message 2" <- w545
                        "Error 2" <- w544
                      }
                    }
                  }
                  frame #2 {
                    w737 = u8 2 items=["1", "2", "3"] ("axis in")
                    n331 = event shown="[7] \"Single Step Left 3\": Value Change" {
                      selector: _ -> [_ _ _ _ _ _ _ _ _ _ _ _ _ _ _ _ _ _]
                      dyn-events: _ -> [_ _ _ _ _ _ _ _ _ _ _ _ _ _ _ _ _ _]
                      timeout: 1 -> [_ _ _ _ _ _ _ _ _ _ _ _ _ _ _ _ _ _]
                      tunnel: w735 -> [w749 w758 w769 w779 w788 w801 w805 w817 w822 w829 w840 w850 _ w863 w873 w878 w887 w917]
                      tunnel: w737 -> [w748 w757 w768 w778 w787 w800 w804 w816 w821 w827 w838 w851 _ w862 w872 w877 w886 w916]
                      tunnel: [w743 w752 w763 w775 w782 w792 w802 w809 w820 w830 w841 w845 _ w857 w867 _ _ w899] -> w733
                      event "amplitude [V] 3": Value Change {
                        n332 = event-data() -> ()  [unwired: 1 in, 1 out]
                        n333 = call "AMC_controlAmplitude.vi"("set"=TRUE, "amplitude [V] in"="amplitude [V] 3", "axis"=w748, "deviceHandle"=w749) -> ("error out"=w744:errorcluster, "axis"=w740:u8, "deviceHandle"=w745:i32)  [unwired: 2 in, 1 out]
                        n334 = call "AMC_controlAmplitude.vi"("set"=FALSE, "error in"=w744, "axis"=w740, "deviceHandle"=w745) -> ("error out"=w743:errorcluster, "amplitude [V] out"=w741:dbl)  [unwired: 2 in, 2 out]
                        n335 = local write "amplitude [V] 3"(w741) -> ()
                      }
                      event "Output 3": Value Change {
                        n336 = event-data() -> ()  [unwired: 1 in, 1 out]
                        n337 = call "AMC_controlOutput.vi"("set"=TRUE, "enable in"="Output 3", "axis"=w757, "deviceHandle"=w758) -> ("error out"=w754:errorcluster, "axis"=w755:u8, "deviceHandle"=w756:i32)  [unwired: 4 in, 1 out]
                        n338 = call "AMC_controlOutput.vi"("set"=FALSE, "error in"=w754, "axis"=w755, "deviceHandle"=w756) -> ("error out"=w752:errorcluster, "enable out"=→"Output Status 3":bool)  [unwired: 4 in, 2 out]
                      }
                      event "frequency [Hz] 3": Value Change {
                        n339 = event-data() -> ()  [unwired: 1 in, 1 out]
                        n340 = call "AMC_controlFrequency.vi"("set"=TRUE, "frequency [Hz] in"="frequency [Hz] 3", "axis"=w768, "deviceHandle"=w769) -> ("error out"=w764:errorcluster, "axis"=w760:u8, "deviceHandle"=w765:i32)  [unwired: 4 in, 1 out]
                        n341 = call "AMC_controlFrequency.vi"("set"=FALSE, "error in"=w764, "axis"=w760, "deviceHandle"=w765) -> ("error out"=w763:errorcluster, "frequency [Hz] out"=w762:dbl)  [unwired: 4 in, 2 out]
                        n342 = local write "frequency [Hz] 3"(w762) -> ()
                      }
                      event "Move 3": Value Change {
                        n343 = event-data() -> ()  [unwired: 1 in, 1 out]
                        n344 = call "AMC_controlMove.vi"("set"=TRUE, "enable in"="Move 3", "axis"=w778, "deviceHandle"=w779) -> ("error out"=w776:errorcluster, "axis"=w773:u8, "deviceHandle"=w774:i32)  [unwired: 4 in, 1 out]
                        n345 = call "AMC_controlMove.vi"("set"=FALSE, "error in"=w776, "axis"=w773, "deviceHandle"=w774) -> ("error out"=w775:errorcluster, "enable out"=→"move out 3":bool)  [unwired: 4 in, 2 out]
                      }
                      event "EoT 3": Value Change {
                        n346 = event-data() -> ()  [unwired: 1 in, 1 out]
                        n347 = call "AMC_controlEotOutputDeactive.vi"("set"=TRUE, "enable in"="EoT 3", "axis"=w787, "deviceHandle"=w788) -> ("error out"=w784:errorcluster, "axis"=w785:u8, "deviceHandle"=w786:i32)  [unwired: 4 in, 1 out]
                        n348 = call "AMC_controlEotOutputDeactive.vi"("set"=FALSE, "error in"=w784, "axis"=w785, "deviceHandle"=w786) -> ("error out"=w782:errorcluster, "enable out"=w780:bool)  [unwired: 4 in, 2 out]
                        n349 = local write "EoT 3"(w780) -> ()
                      }
                      event "Target Position 3": Value Change {
                        n350 = event-data() -> ()  [unwired: 1 in, 1 out]
                        n351 = Multiply(x="Target Position 3", y=1000) -> (x*y=w796:i32)
                        n352 = call "AMC_controlTargetPosition.vi"("set"=TRUE, "target in"=w796, "axis"=w800, "deviceHandle"=w801) -> ("error out"=w793:errorcluster, "axis"=w794:u8, "deviceHandle"=w795:i32)  [unwired: 4 in, 1 out]
                        n353 = call "AMC_controlTargetPosition.vi"("set"=FALSE, "error in"=w793, "axis"=w794, "deviceHandle"=w795) -> ("error out"=w792:errorcluster, "target out"=w790:i32)  [unwired: 4 in, 2 out]
                        n354 = local write "Target Position 3"(w790) -> ()
                      }
                      event "Axis 3": Value Change {
                        n355 = event-data() -> ()  [unwired: 1 in, 1 out]
                        n356 = case shown="True" "Axis 3" {
                          tunnel: w805 -> [_ w807]
                          tunnel: w804 -> [_ w808]
                          tunnel: [_ w806] -> w802
                          frame False {
                          }
                          frame True {
                            n357 = call "AMC_setReset.vi"("axis"=w808, "deviceHandle"=w807) -> ("error out"=w806:errorcluster)  [unwired: 7 in, 2 out]
                          }
                        }
                      }
                      event "Single Step Left 3": Value Change {
                        n358 = event-data() -> ()  [unwired: 1 in, 1 out]
                        n359 = call "AMC_setNSteps.vi"("deviceHandle"=w817, "axis"=w816, "n in"="Number of steps 3", "backwards"=FALSE) -> ("deviceHandle"=w813:i32, "axis"=w812:i32, "error out"=w811:errorcluster)  [unwired: 8 in, 1 out]
                        n360 = call "AMC_getNSteps.vi"("error in"=w811, "axis"=w812, "deviceHandle"=w813) -> ("error out"=w809:errorcluster, "n out"=w810:i32)  [unwired: 5 in, 2 out]
                        n361 = local write "Number of steps 3"(w810) -> ()
                      }
                      event "Single Step Right 3": Value Change {
                        n362 = event-data() -> ()  [unwired: 1 in, 1 out]
                        n363 = local read "Number of steps 3"() -> (w818:i32)
                        n364 = call "AMC_setNSteps.vi"("deviceHandle"=w822, "axis"=w821, "n in"=w818, "backwards"=TRUE) -> ("error out"=w820:errorcluster)  [unwired: 8 in, 3 out]
                      }
                      event "Endless Left 3": Value Change {
                        n365 = event-data() -> ()  [unwired: 1 in, 1 out]
                        n366 = call "AMC_controlContinousFwd.vi"("set"=TRUE, "enable in"=FALSE, "axis"=w827, "deviceHandle"=w829) -> ("axis"=w826:u8, "deviceHandle"=w828:i32)  [unwired: 4 in, 2 out]
                        n367 = call "AMC_controlContinousBkwd.vi"("set"=TRUE, "enable in"="Endless Left 3", "axis"=w826, "deviceHandle"=w828) -> ("error out"=w830:errorcluster)  [unwired: 4 in, 3 out]
                        n368 = local write "Continuous Forward"(FALSE ("Endless Right 3")) -> ()
                      }
                      event "Continuous Forward": Value Change {
                        n369 = event-data() -> ()  [unwired: 1 in, 1 out]
                        n370 = call "AMC_controlContinousBkwd.vi"("set"=TRUE, "enable in"=FALSE, "axis"=w838, "deviceHandle"=w840) -> ("error out"=w836:errorcluster, "axis"=w837:u8, "deviceHandle"=w839:i32)  [unwired: 4 in, 1 out]
                        n371 = call "AMC_controlContinousFwd.vi"("set"=TRUE, "error in"=w836, "enable in"="Continuous Forward", "axis"=w837, "deviceHandle"=w839) -> ("error out"=w841:errorcluster)  [unwired: 3 in, 3 out]
                        n372 = local write "Endless Left 3"(FALSE ("Endless Left 3")) -> ()
                      }
                      event "Fixed DC 3": Value Change {
                        n373 = event-data() -> ()  [unwired: 1 in, 1 out]
                        n374 = call "AMC_controlFixOutputVoltage.vi"("set"=TRUE, "voltage"="Fixed DC 3", "axis"=w851, "deviceHandle"=w850) -> ("error out"=w847:errorcluster, "axis"=w848:u8, "deviceHandle"=w849:i32)  [unwired: 4 in, 1 out]
                        n375 = call "AMC_controlFixOutputVoltage.vi"("set"=FALSE, "error in"=w847, "axis"=w848, "deviceHandle"=w849) -> ("error out"=w845:errorcluster, "voltage"=w844:i32)  [unwired: 4 in, 2 out]
                        n376 = local write "Fixed DC 3"(w844) -> ()
                      }
                      event "Reset Error 3": Value Change {
                        n377 = event-data() -> ()  [unwired: 1 in, 1 out]
                        n378 = local write "Error Message 3"("" ("Error Message 3")) -> ()
                        n379 = local write "Error 3"(FALSE ("Error 3")) -> ()
                      }
                      event "Positioner 3": Value Change {
                        n380 = event-data() -> ()  [unwired: 1 in, 1 out]
                        n381 = property on="Positioner 3" class="Ring (strict)"() -> ("RingText.Text"=w861:string)  [unwired: 2 in, 2 out]
                        n382 = call "AMC_controlActorSelection.vi"("set"=TRUE, "actor in"=w861, "axis"=w862, "deviceHandle"=w863) -> ("error out"=w859:errorcluster, "axis"=w858:u8, "deviceHandle"=w860:i32)  [unwired: 4 in, 1 out]
                        n383 = call "AMC_getActorType.vi"("error in"=w859, "axis"=w858, "deviceHandle"=w860) -> ("error out"=w857:errorcluster, "positioner type"=→"actor type 3":u16)  [unwired: 5 in, 2 out]
                      }
                      event "Target Range 3": Value Change {
                        n384 = event-data() -> ()  [unwired: 1 in, 1 out]
                        n385 = call "AMC_controlTargetRange.vi"("set"=TRUE, "range in"="Target Range 3", "axis"=w872, "deviceHandle"=w873) -> ("error out"=w868:errorcluster, "axis"=w869:u8, "deviceHandle"=w870:i32)  [unwired: 4 in, 1 out]
                        n386 = call "AMC_controlTargetRange.vi"("set"=FALSE, "error in"=w868, "axis"=w869, "deviceHandle"=w870) -> ("error out"=w867:errorcluster, "range out"=w865:u32)  [unwired: 4 in, 2 out]
                        n387 = local write "Target Range 3"(w865) -> ()
                      }
                      event "auto Reset 3": Value Change {
                        n388 = event-data() -> ()  [unwired: 1 in, 1 out]
                        n389 = call "AMC_controlAutoReset.vi"("set"=TRUE, "enable in"="auto Reset 3", "axis"=w877, "deviceHandle in"=w878) -> ("error out"=w880:errorcluster, "axis"=w881:u8, "deviceHandle out"=w882:i32)  [unwired: 4 in, 1 out]
                        n390 = call "AMC_controlAutoReset.vi"("set"=FALSE, "error in"=w880, "axis"=w881, "deviceHandle in"=w882) -> ("enable out"=w875:bool)  [unwired: 4 in, 3 out]
                        n391 = local write "auto Reset 3"(w875) -> ()
                      }
                      event "Reference Auto Update 3": Value Change {
                        n392 = event-data() -> ()  [unwired: 1 in, 1 out]
                        n393 = call "AMC_controlReferenceAutoUpdate.vi"("set"=TRUE, "enable in"="Reference Auto Update 3", "axis"=w886, "deviceHandle"=w887) -> ("error out"=w891:errorcluster, "axis"=w889:u8, "deviceHandle"=w890:i32)  [unwired: 4 in, 1 out]
                        n394 = call "AMC_controlReferenceAutoUpdate.vi"("set"=FALSE, "error in"=w891, "axis"=w889, "deviceHandle"=w890) -> ("enable out"=w884:bool)  [unwired: 4 in, 3 out]
                        n395 = local write "Reference Auto Update 3"(w884) -> ()
                      }
                      event Timeout {
                        n396 = event-data() -> ()  [unwired: 1 in, 1 out]
                        n397 = call "AMC_getPosition.vi"("axis"=w916, "deviceHandle"=w917) -> ("error out"=w915:errorcluster, "position"=→"Position 3":i32, "axis"=w921:u8, "deviceHandle"=w922:i32)  [unwired: 6 in]
                        n398 = call "AMC_getReferencePosition.vi"("error in"=w915, "axis"=w921, "deviceHandle"=w922) -> ("error out"=w905:errorcluster, "reference"=→"Reference 3":i32, "axis"=w907:i32, "deviceHandle"=w909:i32)  [unwired: 5 in]
                        n399 = call "AMC_getStatusConnected.vi"("error in"=w905, "axis"=w907, "deviceHandle"=w909) -> ("error out"=w904:errorcluster, "connected"=→"Connected 3":bool, "axis"=w906:i32, "deviceHandle"=w908:i32)  [unwired: 5 in]
                        n400 = call "AMC_getStatusMoving.vi"("error in"=w904, "axis"=w906, "deviceHandle"=w908) -> ("error out"=w923:errorcluster, "moving"=→"MoveSignal 3":bool, "axis"=w918:i32, "deviceHandle"=w924:i32)  [unwired: 5 in]
                        n401 = call "AMC_getStatusReference.vi"("error in"=w923, "axis"=w918, "deviceHandle"=w924) -> ("error out"=w896:errorcluster, "reference valid"=→"ReferenceSignal 3":bool, "axis"=w897:i32, "deviceHandle"=w898:i32)  [unwired: 5 in]
                        n402 = call "AMC_getStatusEotBkwd.vi"("error in"=w896, "axis"=w897, "deviceHandle"=w898) -> ("error out"=w911:errorcluster, "EotDetected"=→"EotLeftDetected3":bool, "axis"=w913:u8, "deviceHandle"=w912:i32)  [unwired: 5 in]
                        n403 = call "AMC_getStatusEotFwd.vi"("error in"=w911, "axis"=w913, "deviceHandle"=w912) -> ("error out"=w900:errorcluster, "EotDetected"=→"EotrightDetected3":bool, "axis"=w901:u8, "deviceHandle"=w902:i32)  [unwired: 5 in]
                        n404 = call "AMC_getStatusTargetRange.vi"("error in"=w900, "axis"=w901, "deviceHandle"=w902) -> ("error out"=w899:errorcluster, "in target range"=→"in target range3":bool)  [unwired: 5 in, 2 out]
                      }
                    }
                    n405 = Unbundle(w733) -> ("code"=w732:i32, "source"=w734:string)  [unwired: 1 out]
                    n406 = Not Equal To 0?(x=w732) -> (x != 0?=w731:bool)
                    n407 = case shown="True" w731 {
                      selector: w731 -> [_ w738]
                      tunnel: w734 -> [_ w739]
                      frame False {
                      }
                      frame True {
                        "Error Message 3" <- w739
                        "Error 3" <- w738
                      }
                    }
                  }
                }
              }
              frame "Interface" {
                n408 = stacked-sequence {
                  tunnel: w925 -> [w932 w1056 w1179]
                  frame #0 {
                    w931 = u8 0 items=["1", "2", "3"] ("axis in")
                    n409 = event shown="[4] \"Change per pulse 1\": Value Change" {
                      selector: _ -> [_ _ _ _ _ _ _ _ _ _ _]
                      dyn-events: _ -> [_ _ _ _ _ _ _ _ _ _ _]
                      timeout: 1 -> [_ _ _ _ _ _ _ _ _ _ _]
                      tunnel: w932 -> [w944 w967 w977 w988 w998 w1008 w1016 w1027 w1038 w1047 _]
                      tunnel: w931 -> [w942 w966 w976 w987 w997 w1007 w1015 w1028 w1037 w1044 _]
                      tunnel: [_ w954 w969 w978 w993 w1001 w1010 w1021 w1033 w1040 _] -> w928
                      event Timeout {
                        n410 = event-data() -> ()  [unwired: 1 in, 1 out]
                        n411 = call "AMC_controlRealtimeInputMode.vi"("set"=FALSE, "axis"=w942, "deviceHandle"=w944) -> ("mode out"=w936:i32, "axis"=w941:u8, "deviceHandle"=w943:i32)  [unwired: 5 in, 1 out]
                        n412 = local write "Mode Input 1"(w936) -> ()
                        n413 = Equal?(x=w936, y=15) -> (x = y?=w939:bool)
                        n414 = call "AMC_controlRealtimeInputLoopMode.vi"("set"=FALSE, "axis"=w941, "deviceHandle"=w943) -> ("mode out"=w935:i32)  [unwired: 5 in, 3 out]
                        n415 = local write "Loop Mode 1"(w935) -> ()
                        n416 = Equal?(x=w935, y=0) -> (x = y?=w937:bool)
                        n417 = case shown="False" w939 {
                          tunnel: w937 -> [w947 _]
                          frame False {
                            n418 = case shown="True" w947 {
                              frame False {
                                w948 = T1."Enabled" ("Disabled")
                                n419 = property on="RT in move 1" class="Bool (strict)"("DisabledEnum"=w948) -> ()  [unwired: 2 in, 2 out]
                                n420 = property on="RT in move Signal 1" class="Bool (strict)"("DisabledEnum"=w948) -> ()  [unwired: 2 in, 2 out]
                                n421 = property on="Loop Mode 1" class="Ring (strict)"("DisabledEnum"=w948) -> ()  [unwired: 2 in, 2 out]
                                n422 = property on="Steps per pulse 1" class="DigNum (strict)"("DisabledEnum"=T1."Disabled and Grayed Out" ("Disabled")) -> ()  [unwired: 2 in, 2 out]
                                n423 = property on="Change per pulse 1" class="DigNum (strict)"("DisabledEnum"=w948) -> ()  [unwired: 2 in, 2 out]
                              }
                              frame True {
                                w951 = T1."Enabled" ("Disabled")
                                w950 = T1."Disabled and Grayed Out" ("Disabled")
                                n424 = property on="RT in move 1" class="Bool (strict)"("DisabledEnum"=w950) -> ()  [unwired: 2 in, 2 out]
                                n425 = property on="RT in move Signal 1" class="Bool (strict)"("DisabledEnum"=w950) -> ()  [unwired: 2 in, 2 out]
                                n426 = property on="Loop Mode 1" class="Ring (strict)"("DisabledEnum"=w951) -> ()  [unwired: 2 in, 2 out]
                                n427 = property on="Steps per pulse 1" class="DigNum (strict)"("DisabledEnum"=w951) -> ()  [unwired: 2 in, 2 out]
                                n428 = property on="Change per pulse 1" class="DigNum (strict)"("DisabledEnum"=w950) -> ()  [unwired: 2 in, 2 out]
                              }
                            }
                          }
                          frame True {
                            w952 = T1."Disabled and Grayed Out" ("Disabled")
                            n429 = property on="RT in move 1" class="Bool (strict)"("DisabledEnum"=w952) -> ()  [unwired: 2 in, 2 out]
                            n430 = property on="RT in move Signal 1" class="Bool (strict)"("DisabledEnum"=w952) -> ()  [unwired: 2 in, 2 out]
                            n431 = property on="Loop Mode 1" class="Ring (strict)"("DisabledEnum"=w952) -> ()  [unwired: 2 in, 2 out]
                            n432 = property on="Steps per pulse 1" class="DigNum (strict)"("DisabledEnum"=w952) -> ()  [unwired: 2 in, 2 out]
                            n433 = property on="Change per pulse 1" class="DigNum (strict)"("DisabledEnum"=w952) -> ()  [unwired: 2 in, 2 out]
                          }
                        }
                      }
                      event "Mode Input 1": Value Change {
                        n434 = event-data() -> ()  [unwired: 1 in, 1 out]
                        n435 = call "AMC_controlRealtimeInputMode.vi"("set"=TRUE, "mode in"="Mode Input 1", "axis"=w966, "deviceHandle"=w967) -> ("error out"=w961:errorcluster, "axis"=w962:u8, "deviceHandle"=w963:i32)  [unwired: 4 in, 1 out]
                        n436 = call "AMC_controlRealtimeInputMode.vi"("set"=FALSE, "error in"=w961, "axis"=w962, "deviceHandle"=w963) -> ("error out"=w955:errorcluster, "mode out"=w959:i32, "axis"=w956:u8, "deviceHandle"=w957:i32)  [unwired: 4 in]
                        n437 = local write "Mode Input 1"(w959) -> ()
                        n438 = call "AMC_controlRealtimeInputLoopMode.vi"("set"=FALSE, "error in"=w955, "axis"=w956, "deviceHandle"=w957) -> ("error out"=w954:errorcluster, "mode out"=w953:i32)  [unwired: 4 in, 2 out]
                        n439 = local write "Loop Mode 1"(w953) -> ()
                      }
                      event "Loop Mode 1": Value Change {
                        n440 = event-data() -> ()  [unwired: 1 in, 1 out]
                        n441 = call "AMC_controlRealtimeInputLoopMode.vi"("set"=TRUE, "mode in"="Loop Mode 1", "axis"=w976, "deviceHandle"=w977) -> ("error out"=w970:errorcluster, "axis"=w974:u8, "deviceHandle"=w975:i32)  [unwired: 4 in, 1 out]
                        n442 = call "AMC_controlRealtimeInputLoopMode.vi"("set"=FALSE, "error in"=w970, "axis"=w974, "deviceHandle"=w975) -> ("error out"=w969:errorcluster, "mode out"=w968:i32)  [unwired: 4 in, 2 out]
                        n443 = local write "Loop Mode 1"(w968) -> ()
                      }
                      event "Steps per pulse 1": Value Change {
                        n444 = event-data() -> ()  [unwired: 1 in, 1 out]
                        n445 = call "AMC_controlRealtimeInputStepsPerPulse.vi"("set"=TRUE, "steps in"="Steps per pulse 1", "axis"=w987, "deviceHandle"=w988) -> ("error out"=w979:errorcluster, "axis"=w985:u8, "deviceHandle"=w986:i32)  [unwired: 4 in, 1 out]
                        n446 = call "AMC_controlRealtimeInputStepsPerPulse.vi"("set"=FALSE, "axis"=w985, "deviceHandle"=w986) -> ("error out"=w980:errorcluster, "steps out"=w981:i32)  [unwired: 5 in, 2 out]
                        n447 = local write "Steps per pulse 1"(w981) -> ()
                        n448 = Merge Errors(w980, w979) -> (w978:errorcluster)
                      }
                      event "Change per pulse 1": Value Change {
                        n449 = event-data() -> ()  [unwired: 1 in, 1 out]
                        n450 = call "AMC_controlRealtimeInputChangePerPulse.vi"("set"=TRUE, "change in"="Change per pulse 1", "axis"=w997, "deviceHandle"=w998) -> ("error out"=w994:errorcluster, "axis"=w995:u8, "deviceHandle"=w996:i32)  [unwired: 4 in, 1 out]
                        n451 = call "AMC_controlRealtimeInputChangePerPulse.vi"("set"=FALSE, "error in"=w994, "axis"=w995, "deviceHandle"=w996) -> ("error out"=w993:errorcluster, "change out"=w989:i32)  [unwired: 4 in, 2 out]
                        n452 = local write "Change per pulse 1"(w989) -> ()
                      }
                      event "RT in move 1": Value Change {
                        n453 = event-data() -> ()  [unwired: 1 in, 1 out]
                        n454 = call "AMC_controlRealtimeInputMove.vi"("set"=TRUE, "enable in"="RT in move 1", "axis"=w1007, "deviceHandle"=w1008) -> ("error out"=w1002:errorcluster, "axis"=w1003:u8, "deviceHandle"=w1004:i32)  [unwired: 4 in, 1 out]
                        n455 = call "AMC_controlRealtimeInputMove.vi"("set"=FALSE, "error in"=w1002, "axis"=w1003, "deviceHandle"=w1004) -> ("error out"=w1001:errorcluster, "enable out"=→"RT in move Signal 1":bool)  [unwired: 4 in, 2 out]
                      }
                      event "AquadB in res 1": Value Change {
                        n456 = event-data() -> ()  [unwired: 1 in, 1 out]
                        n457 = call "AMC_controlAQuadBInResolution.vi"("set"=TRUE, "resolution in"="AquadB in res 1", "axis"=w1015, "deviceHandle"=w1016) -> ("error out"=w1012:errorcluster, "axis"=w1013:u8, "deviceHandle"=w1014:i32)  [unwired: 4 in, 1 out]
                        n458 = call "AMC_controlAQuadBInResolution.vi"("set"=FALSE, "error in"=w1012, "axis"=w1013, "deviceHandle"=w1014) -> ("error out"=w1010:errorcluster, "resolution out"=w1009:i32)  [unwired: 4 in, 2 out]
                        n459 = local write "AquadB in res 1"(w1009) -> ()
                      }
                      event "AquadB out 1": Value Change {
                        n460 = event-data() -> ()  [unwired: 1 in, 1 out]
                        n461 = call "AMC_controlAQuadBOut.vi"("set"=TRUE, "enable in"="AquadB out 1", "axis"=w1028, "deviceHandle"=w1027) -> ("error out"=w1022:errorcluster, "axis"=w1023:u8, "deviceHandle"=w1024:i32)  [unwired: 4 in, 1 out]
                        n462 = call "AMC_controlAQuadBOut.vi"("set"=FALSE, "error in"=w1022, "axis"=w1023, "deviceHandle"=w1024) -> ("error out"=w1021:errorcluster, "enable out"=w1019:bool)  [unwired: 4 in, 2 out]
                        n463 = local write "AquadB out 1"(w1019) -> ()
                      }
                      event "AqaudB clock 1": Value Change {
                        (unwired) TRUE ("set")
                        n464 = event-data() -> ()  [unwired: 1 in, 1 out]
                        n465 = call "AMC_controlAQuadBOutClock.vi"("set"=TRUE, "clock in"="AqaudB clock 1", "axis"=w1037, "deviceHandle"=w1038) -> ("error out"=w1034:errorcluster, "axis"=w1030:u8, "deviceHandle"=w1031:i32)  [unwired: 4 in, 1 out]
                        n466 = call "AMC_controlAQuadBOutClock.vi"("set"=FALSE, "error in"=w1034, "axis"=w1030, "deviceHandle"=w1031) -> ("error out"=w1033:errorcluster, "clock out"=w1032:i32)  [unwired: 4 in, 2 out]
                        n467 = local write "AqaudB clock 1"(w1032) -> ()
                      }
                      event "AquadB Resolution 1": Value Change {
                        n468 = event-data() -> ()  [unwired: 1 in, 1 out]
                        n469 = call "AMC_controlAQuadBOutResolution.vi"("set"=TRUE, "resolution in"="AquadB Resolution 1", "axis"=w1044, "deviceHandle"=w1047) -> ("axis"=w1041:u8, "deviceHandle"=w1042:i32)  [unwired: 4 in, 2 out]
                        n470 = call "AMC_controlAQuadBOutResolution.vi"("set"=FALSE, "axis"=w1041, "deviceHandle"=w1042) -> ("error out"=w1040:errorcluster, "resolution out"=w1039:i32)  [unwired: 5 in, 2 out]
                        n471 = local write "AquadB Resolution 1"(w1039) -> ()
                      }
                      event "Reset Error 4": Value Change {
                        n472 = event-data() -> ()  [unwired: 1 in, 1 out]
                        n473 = local write "Error Message 4"("" ("Error Message")) -> ()
                        n474 = local write "Error 4"(FALSE ("Error 4")) -> ()
                      }
                    }
                    n475 = Unbundle(w928) -> ("code"=w926:i32, "source"=w927:string)  [unwired: 1 out]
                    n476 = Not Equal To 0?(x=w926) -> (x != 0?=w929:bool)
                    n477 = case shown="True" w929 {
                      selector: w929 -> [_ w933]
                      tunnel: w927 -> [_ w934]
                      frame False {
                      }
                      frame True {
                        "Error Message 4" <- w934
                        "Error 4" <- w933
                      }
                    }
                  }
                  frame #1 {
                    w1055 = u8 1 items=["1", "2", "3"] ("axis in")
                    n478 = event shown="[4] \"Change per pulse 2\": Value Change" {
                      selector: _ -> [_ _ _ _ _ _ _ _ _ _ _]
                      dyn-events: _ -> [_ _ _ _ _ _ _ _ _ _ _]
                      timeout: 1 -> [_ _ _ _ _ _ _ _ _ _ _]
                      tunnel: w1056 -> [w1062 w1087 w1096 w1107 w1116 w1126 w1139 w1150 w1160 w1170 _]
                      tunnel: w1055 -> [w1061 w1085 w1093 w1104 w1115 w1124 w1138 w1151 w1159 w1169 _]
                      tunnel: [_ w1078 w1095 w1105 w1114 w1122 w1133 w1144 w1153 w1163 _] -> w1050
                      event Timeout {
                        n479 = event-data() -> ()  [unwired: 1 in, 1 out]
                        n480 = call "AMC_controlRealtimeInputMode.vi"("set"=FALSE, "axis"=w1061, "deviceHandle"=w1062) -> ("mode out"=w1060:i32, "axis"=w1067:u8, "deviceHandle"=w1068:i32)  [unwired: 5 in, 1 out]
                        n481 = local write "Mode Input 2"(w1060) -> ()
                        n482 = Equal?(x=w1060, y=15) -> (x = y?=w1065:bool)
                        n483 = call "AMC_controlRealtimeInputLoopMode.vi"("set"=FALSE, "axis"=w1067, "deviceHandle"=w1068) -> ("mode out"=w1059:i32)  [unwired: 5 in, 3 out]
                        n484 = local write "Loop Mode 2"(w1059) -> ()
                        n485 = Equal?(x=w1059, y=0) -> (x = y?=w1063:bool)
                        n486 = case shown="False" w1065 {
                          tunnel: w1063 -> [w1071 _]
                          frame False {
                            n487 = case shown="False" w1071 {
                              frame False {
                                w1072 = T1."Enabled" ("Disabled")
                                n488 = property on="RT in move 2" class="Bool (strict)"("DisabledEnum"=w1072) -> ()  [unwired: 2 in, 2 out]
                                n489 = property on="RT in move Signal 2" class="Bool (strict)"("DisabledEnum"=w1072) -> ()  [unwired: 2 in, 2 out]
                                n490 = property on="Loop Mode 2" class="Ring (strict)"("DisabledEnum"=w1072) -> ()  [unwired: 2 in, 2 out]
                                n491 = property on="Steps per pulse 2" class="DigNum (strict)"("DisabledEnum"=T1."Disabled and Grayed Out" ("Disabled")) -> ()  [unwired: 2 in, 2 out]
                                n492 = property on="Change per pulse 2" class="DigNum (strict)"("DisabledEnum"=w1072) -> ()  [unwired: 2 in, 2 out]
                              }
                              frame True {
                                w1075 = T1."Enabled" ("Disabled")
                                w1074 = T1."Disabled and Grayed Out" ("Disabled")
                                n493 = property on="RT in move 2" class="Bool (strict)"("DisabledEnum"=w1074) -> ()  [unwired: 2 in, 2 out]
                                n494 = property on="RT in move Signal 2" class="Bool (strict)"("DisabledEnum"=w1074) -> ()  [unwired: 2 in, 2 out]
                                n495 = property on="Loop Mode 2" class="Ring (strict)"("DisabledEnum"=w1075) -> ()  [unwired: 2 in, 2 out]
                                n496 = property on="Steps per pulse 2" class="DigNum (strict)"("DisabledEnum"=w1075) -> ()  [unwired: 2 in, 2 out]
                                n497 = property on="Change per pulse 2" class="DigNum (strict)"("DisabledEnum"=w1074) -> ()  [unwired: 2 in, 2 out]
                              }
                            }
                          }
                          frame True {
                            w1076 = T1."Disabled and Grayed Out" ("Disabled")
                            n498 = property on="RT in move 2" class="Bool (strict)"("DisabledEnum"=w1076) -> ()  [unwired: 2 in, 2 out]
                            n499 = property on="RT in move Signal 2" class="Bool (strict)"("DisabledEnum"=w1076) -> ()  [unwired: 2 in, 2 out]
                            n500 = property on="Loop Mode 2" class="Ring (strict)"("DisabledEnum"=w1076) -> ()  [unwired: 2 in, 2 out]
                            n501 = property on="Steps per pulse 2" class="DigNum (strict)"("DisabledEnum"=w1076) -> ()  [unwired: 2 in, 2 out]
                            n502 = property on="Change per pulse 2" class="DigNum (strict)"("DisabledEnum"=w1076) -> ()  [unwired: 2 in, 2 out]
                          }
                        }
                      }
                      event "Mode Input 2": Value Change {
                        n503 = event-data() -> ()  [unwired: 1 in, 1 out]
                        n504 = call "AMC_controlRealtimeInputMode.vi"("set"=TRUE, "mode in"="Mode Input 2", "axis"=w1085, "deviceHandle"=w1087) -> ("error out"=w1083:errorcluster, "axis"=w1089:u8, "deviceHandle"=w1090:i32)  [unwired: 4 in, 1 out]
                        n505 = call "AMC_controlRealtimeInputMode.vi"("set"=FALSE, "error in"=w1083, "axis"=w1089, "deviceHandle"=w1090) -> ("error out"=w1079:errorcluster, "mode out"=w1084:i32, "axis"=w1080:u8, "deviceHandle"=w1081:i32)  [unwired: 4 in]
                        n506 = local write "Mode Input 2"(w1084) -> ()
                        n507 = call "AMC_controlRealtimeInputLoopMode.vi"("set"=FALSE, "error in"=w1079, "axis"=w1080, "deviceHandle"=w1081) -> ("error out"=w1078:errorcluster, "mode out"=w1077:i32)  [unwired: 4 in, 2 out]
                        n508 = local write "Loop Mode 2"(w1077) -> ()
                      }
                      event "Loop Mode 2": Value Change {
                        n509 = event-data() -> ()  [unwired: 1 in, 1 out]
                        n510 = call "AMC_controlRealtimeInputLoopMode.vi"("set"=TRUE, "mode in"="Loop Mode 2", "axis"=w1093, "deviceHandle"=w1096) -> ("error out"=w1097:errorcluster, "axis"=w1100:u8, "deviceHandle"=w1101:i32)  [unwired: 4 in, 1 out]
                        n511 = call "AMC_controlRealtimeInputLoopMode.vi"("set"=FALSE, "error in"=w1097, "axis"=w1100, "deviceHandle"=w1101) -> ("error out"=w1095:errorcluster, "mode out"=w1092:i32)  [unwired: 4 in, 2 out]
                        n512 = local write "Loop Mode 2"(w1092) -> ()
                      }
                      event "Steps per pulse 2": Value Change {
                        n513 = event-data() -> ()  [unwired: 1 in, 1 out]
                        n514 = call "AMC_controlRealtimeInputStepsPerPulse.vi"("set"=TRUE, "steps in"="Steps per pulse 2", "axis"=w1104, "deviceHandle"=w1107) -> ("error out"=w1106:errorcluster, "axis"=w1110:u8, "deviceHandle"=w1111:i32)  [unwired: 4 in, 1 out]
                        n515 = call "AMC_controlRealtimeInputStepsPerPulse.vi"("set"=FALSE, "error in"=w1106, "axis"=w1110, "deviceHandle"=w1111) -> ("error out"=w1105:errorcluster, "steps out"=w1102:i32)  [unwired: 4 in, 2 out]
                        n516 = local write "Steps per pulse 2"(w1102) -> ()
                      }
                      event "Change per pulse 2": Value Change {
                        n517 = event-data() -> ()  [unwired: 1 in, 1 out]
                        n518 = call "AMC_controlRealtimeInputChangePerPulse.vi"("set"=TRUE, "change in"="Change per pulse 2", "axis"=w1115, "deviceHandle"=w1116) -> ("error out"=w1119:errorcluster, "axis"=w1120:u8, "deviceHandle"=w1121:i32)  [unwired: 4 in, 1 out]
                        n519 = call "AMC_controlRealtimeInputChangePerPulse.vi"("set"=FALSE, "error in"=w1119, "axis"=w1120, "deviceHandle"=w1121) -> ("error out"=w1114:errorcluster, "change out"=w1112:i32)  [unwired: 4 in, 2 out]
                        n520 = local write "Change per pulse 2"(w1112) -> ()
                      }
                      event "RT in move 2": Value Change {
                        n521 = event-data() -> ()  [unwired: 1 in, 1 out]
                        n522 = call "AMC_controlRealtimeInputMove.vi"("set"=TRUE, "enable in"="RT in move 2", "axis"=w1124, "deviceHandle"=w1126) -> ("error out"=w1128:errorcluster, "axis"=w1129:u8, "deviceHandle"=w1130:i32)  [unwired: 4 in, 1 out]
                        n523 = call "AMC_controlRealtimeInputMove.vi"("set"=FALSE, "error in"=w1128, "axis"=w1129, "deviceHandle"=w1130) -> ("error out"=w1122:errorcluster, "enable out"=→"RT in move Signal 2":bool)  [unwired: 4 in, 2 out]
                      }
                      event "AquadB in res 2": Value Change {
                        n524 = event-data() -> ()  [unwired: 1 in, 1 out]
                        n525 = call "AMC_controlAQuadBInResolution.vi"("set"=TRUE, "resolution in"="AquadB in res 2", "axis"=w1138, "deviceHandle"=w1139) -> ("error out"=w1135:errorcluster, "axis"=w1136:u8, "deviceHandle"=w1137:i32)  [unwired: 4 in, 1 out]
                        n526 = call "AMC_controlAQuadBInResolution.vi"("set"=FALSE, "error in"=w1135, "axis"=w1136, "deviceHandle"=w1137) -> ("error out"=w1133:errorcluster, "resolution out"=w1132:i32)  [unwired: 4 in, 2 out]
                        n527 = local write "AquadB in res 2"(w1132) -> ()
                      }
                      event "AquadB out 2": Value Change {
                        n528 = event-data() -> ()  [unwired: 1 in, 1 out]
                        n529 = call "AMC_controlAQuadBOut.vi"("set"=TRUE, "enable in"="AquadB out 2", "axis"=w1151, "deviceHandle"=w1150) -> ("error out"=w1145:errorcluster, "axis"=w1146:u8, "deviceHandle"=w1147:i32)  [unwired: 4 in, 1 out]
                        n530 = call "AMC_controlAQuadBOut.vi"("set"=FALSE, "error in"=w1145, "axis"=w1146, "deviceHandle"=w1147) -> ("error out"=w1144:errorcluster, "enable out"=w1142:bool)  [unwired: 4 in, 2 out]
                        n531 = local write "AquadB out 2"(w1142) -> ()
                      }
                      event "AqaudB clock 2": Value Change {
                        n532 = event-data() -> ()  [unwired: 1 in, 1 out]
                        n533 = call "AMC_controlAQuadBOutClock.vi"("set"=TRUE, "clock in"="AqaudB clock 2", "axis"=w1159, "deviceHandle"=w1160) -> ("error out"=w1154:errorcluster, "axis"=w1155:u8, "deviceHandle"=w1156:i32)  [unwired: 4 in, 1 out]
                        n534 = call "AMC_controlAQuadBOutClock.vi"("set"=FALSE, "error in"=w1154, "axis"=w1155, "deviceHandle"=w1156) -> ("error out"=w1153:errorcluster, "clock out"=w1152:i32)  [unwired: 4 in, 2 out]
                        n535 = local write "AqaudB clock 2"(w1152) -> ()
                      }
                      event "AquadB Resolution 2": Value Change {
                        n536 = event-data() -> ()  [unwired: 1 in, 1 out]
                        n537 = call "AMC_controlAQuadBOutResolution.vi"("set"=TRUE, "resolution in"="AquadB Resolution 2", "axis"=w1169, "deviceHandle"=w1170) -> ("error out"=w1164:errorcluster, "axis"=w1165:u8, "deviceHandle"=w1166:i32)  [unwired: 4 in, 1 out]
                        n538 = call "AMC_controlAQuadBOutResolution.vi"("set"=FALSE, "error in"=w1164, "axis"=w1165, "deviceHandle"=w1166) -> ("error out"=w1163:errorcluster, "resolution out"=w1162:i32)  [unwired: 4 in, 2 out]
                        n539 = local write "AquadB Resolution 2"(w1162) -> ()
                      }
                      event "Reset Error 5": Value Change {
                        n540 = event-data() -> ()  [unwired: 1 in, 1 out]
                        n541 = local write "Error 5"(FALSE ("Error 5")) -> ()
                        n542 = local write "Error Message 5"("" ("Error Message")) -> ()
                      }
                    }
                    n543 = Unbundle(w1050) -> ("code"=w1052:i32, "source"=w1051:string)  [unwired: 1 out]
                    n544 = Not Equal To 0?(x=w1052) -> (x != 0?=w1053:bool)
                    n545 = case shown="True" w1053 {
                      selector: w1053 -> [_ w1057]
                      tunnel: w1051 -> [_ w1058]
                      frame False {
                      }
                      frame True {
                        "Error Message 5" <- w1058
                        "Error 5" <- w1057
                      }
                    }
                  }
                  frame #2 {
                    w1178 = u8 2 items=["1", "2", "3"] ("axis in")
                    n546 = event shown="[4] \"Change per pulse 3\": Value Change" {
                      selector: _ -> [_ _ _ _ _ _ _ _ _ _ _ _]
                      dyn-events: _ -> [_ _ _ _ _ _ _ _ _ _ _ _]
                      timeout: 1 -> [_ _ _ _ _ _ _ _ _ _ _ _]
                      tunnel: w1179 -> [w1186 w1210 w1220 w1230 w1240 w1250 w1263 w1272 w1283 w1292 w1302 _]
                      tunnel: w1178 -> [w1185 w1209 w1218 w1229 w1238 w1249 w1262 _ w1284 w1291 w1301 _]
                      tunnel: [_ w1202 w1219 w1227 w1239 w1248 w1258 w1268 w1277 w1286 w1296 _] -> w1174
                      event Timeout {
                        n547 = event-data() -> ()  [unwired: 1 in, 1 out]
                        n548 = call "AMC_controlRealtimeInputMode.vi"("set"=FALSE, "axis"=w1185, "deviceHandle"=w1186) -> ("mode out"=w1184:i32, "axis"=w1191:u8, "deviceHandle"=w1192:i32)  [unwired: 5 in, 1 out]
                        n549 = local write "Mode Input 3"(w1184) -> ()
                        n550 = Equal?(x=w1184, y=15) -> (x = y?=w1189:bool)
                        n551 = call "AMC_controlRealtimeInputLoopMode.vi"("set"=FALSE, "axis"=w1191, "deviceHandle"=w1192) -> ("mode out"=w1183:i32)  [unwired: 5 in, 3 out]
                        n552 = local write "Loop Mode 3"(w1183) -> ()
                        n553 = Equal?(x=w1183, y=0) -> (x = y?=w1187:bool)
                        n554 = case shown="False" w1189 {
                          tunnel: w1187 -> [w1195 _]
                          frame False {
                            n555 = case shown="True" w1195 {
                              frame False {
                                w1196 = T1."Enabled" ("Disabled")
                                n556 = property on="RT in move 3" class="Bool (strict)"("DisabledEnum"=w1196) -> ()  [unwired: 2 in, 2 out]
                                n557 = property on="RT in move Signal 3" class="Bool (strict)"("DisabledEnum"=w1196) -> ()  [unwired: 2 in, 2 out]
                                n558 = property on="Loop Mode 3" class="Ring (strict)"("DisabledEnum"=w1196) -> ()  [unwired: 2 in, 2 out]
                                n559 = property on="Steps per pulse 3" class="DigNum (strict)"("DisabledEnum"=T1."Disabled and Grayed Out" ("Disabled")) -> ()  [unwired: 2 in, 2 out]
                                n560 = property on="Change per pulse 3" class="DigNum (strict)"("DisabledEnum"=w1196) -> ()  [unwired: 2 in, 2 out]
                              }
                              frame True {
                                w1199 = T1."Enabled" ("Disabled")
                                w1198 = T1."Disabled and Grayed Out" ("Disabled")
                                n561 = property on="RT in move 3" class="Bool (strict)"("DisabledEnum"=w1198) -> ()  [unwired: 2 in, 2 out]
                                n562 = property on="RT in move Signal 3" class="Bool (strict)"("DisabledEnum"=w1198) -> ()  [unwired: 2 in, 2 out]
                                n563 = property on="Loop Mode 3" class="Ring (strict)"("DisabledEnum"=w1199) -> ()  [unwired: 2 in, 2 out]
                                n564 = property on="Steps per pulse 3" class="DigNum (strict)"("DisabledEnum"=w1199) -> ()  [unwired: 2 in, 2 out]
                                n565 = property on="Change per pulse 3" class="DigNum (strict)"("DisabledEnum"=w1198) -> ()  [unwired: 2 in, 2 out]
                              }
                            }
                          }
                          frame True {
                            w1200 = T1."Disabled and Grayed Out" ("Disabled")
                            n566 = property on="RT in move 3" class="Bool (strict)"("DisabledEnum"=w1200) -> ()  [unwired: 2 in, 2 out]
                            n567 = property on="RT in move Signal 3" class="Bool (strict)"("DisabledEnum"=w1200) -> ()  [unwired: 2 in, 2 out]
                            n568 = property on="Loop Mode 3" class="Ring (strict)"("DisabledEnum"=w1200) -> ()  [unwired: 2 in, 2 out]
                            n569 = property on="Steps per pulse 3" class="DigNum (strict)"("DisabledEnum"=w1200) -> ()  [unwired: 2 in, 2 out]
                            n570 = property on="Change per pulse 3" class="DigNum (strict)"("DisabledEnum"=w1200) -> ()  [unwired: 2 in, 2 out]
                          }
                        }
                      }
                      event "Mode Input 3": Value Change {
                        n571 = event-data() -> ()  [unwired: 1 in, 1 out]
                        n572 = call "AMC_controlRealtimeInputMode.vi"("set"=TRUE, "mode in"="Mode Input 3", "axis"=w1209, "deviceHandle"=w1210) -> ("error out"=w1212:errorcluster, "axis"=w1213:u8, "deviceHandle"=w1214:i32)  [unwired: 4 in, 1 out]
                        n573 = call "AMC_controlRealtimeInputMode.vi"("set"=FALSE, "error in"=w1212, "axis"=w1213, "deviceHandle"=w1214) -> ("error out"=w1203:errorcluster, "mode out"=w1207:i32, "axis"=w1204:u8, "deviceHandle"=w1205:i32)  [unwired: 4 in]
                        n574 = local write "Mode Input 3"(w1207) -> ()
                        n575 = call "AMC_controlRealtimeInputLoopMode.vi"("set"=FALSE, "error in"=w1203, "axis"=w1204, "deviceHandle"=w1205) -> ("error out"=w1202:errorcluster, "mode out"=w1201:i32)  [unwired: 4 in, 2 out]
                        n576 = local write "Loop Mode 3"(w1201) -> ()
                      }
                      event "Loop Mode 3": Value Change {
                        n577 = event-data() -> ()  [unwired: 1 in, 1 out]
                        n578 = call "AMC_controlRealtimeInputLoopMode.vi"("set"=TRUE, "mode in"="Loop Mode 3", "axis"=w1218, "deviceHandle"=w1220) -> ("error out"=w1225:errorcluster, "axis"=w1222:u8, "deviceHandle"=w1221:i32)  [unwired: 4 in, 1 out]
                        n579 = call "AMC_controlRealtimeInputLoopMode.vi"("set"=FALSE, "error in"=w1225, "axis"=w1222, "deviceHandle"=w1221) -> ("error out"=w1219:errorcluster, "mode out"=w1216:i32)  [unwired: 4 in, 2 out]
                        n580 = local write "Loop Mode 3"(w1216) -> ()
                      }
                      event "Steps per pulse 3": Value Change {
                        n581 = event-data() -> ()  [unwired: 1 in, 1 out]
                        n582 = call "AMC_controlRealtimeInputStepsPerPulse.vi"("set"=TRUE, "steps in"="Steps per pulse 3", "axis"=w1229, "deviceHandle"=w1230) -> ("error out"=w1235:errorcluster, "axis"=w1232:u8, "deviceHandle"=w1231:i32)  [unwired: 4 in, 1 out]
                        n583 = call "AMC_controlRealtimeInputStepsPerPulse.vi"("set"=FALSE, "error in"=w1235, "axis"=w1232, "deviceHandle"=w1231) -> ("error out"=w1227:errorcluster, "steps out"=w1226:i32)  [unwired: 4 in, 2 out]
                        n584 = local write "Steps per pulse 3"(w1226) -> ()
                      }
                      event "Change per pulse 3": Value Change {
                        n585 = event-data() -> ()  [unwired: 1 in, 1 out]
                        n586 = call "AMC_controlRealtimeInputChangePerPulse.vi"("set"=TRUE, "change in"="Change per pulse 3", "axis"=w1238, "deviceHandle"=w1240) -> ("error out"=w1243:errorcluster, "axis"=w1242:u8, "deviceHandle"=w1241:i32)  [unwired: 4 in, 1 out]
                        n587 = call "AMC_controlRealtimeInputChangePerPulse.vi"("set"=FALSE, "error in"=w1243, "axis"=w1242, "deviceHandle"=w1241) -> ("error out"=w1239:errorcluster, "change out"=w1236:i32)  [unwired: 4 in, 2 out]
                        n588 = local write "Change per pulse 3"(w1236) -> ()
                      }
                      event "RT in move 3": Value Change {
                        n589 = event-data() -> ()  [unwired: 1 in, 1 out]
                        n590 = call "AMC_controlRealtimeInputMove.vi"("set"=TRUE, "enable in"="RT in move 3", "axis"=w1249, "deviceHandle"=w1250) -> ("error out"=w1254:errorcluster, "axis"=w1253:u8, "deviceHandle"=w1252:i32)  [unwired: 4 in, 1 out]
                        n591 = call "AMC_controlRealtimeInputMove.vi"("set"=FALSE, "error in"=w1254, "axis"=w1253, "deviceHandle"=w1252) -> ("error out"=w1248:errorcluster, "enable out"=→"RT in move Signal 3":bool)  [unwired: 4 in, 2 out]
                      }
                      event "AquadB in res 3": Value Change {
                        n592 = event-data() -> ()  [unwired: 1 in, 1 out]
                        n593 = call "AMC_controlAQuadBInResolution.vi"("set"=TRUE, "resolution in"="AquadB in res 3", "axis"=w1262, "deviceHandle"=w1263) -> ("error out"=w1259:errorcluster, "axis"=w1260:u8, "deviceHandle"=w1261:i32)  [unwired: 4 in, 1 out]
                        n594 = call "AMC_controlAQuadBInResolution.vi"("set"=FALSE, "error in"=w1259, "axis"=w1260, "deviceHandle"=w1261) -> ("error out"=w1258:errorcluster, "resolution out"=w1256:i32)  [unwired: 4 in, 2 out]
                        n595 = local write "AquadB in res 3"(w1256) -> ()
                      }
                      event "Output Mode": Value Change {
                        n596 = event-data() -> ()  [unwired: 1 in, 1 out]
                        n597 = call "AMC_controlRtOutSignalMode.vi"("deviceHandle"=w1272, "mode in"="Output Mode", "set"=TRUE) -> ("deviceHandle"=w1271:i32, "mode out"=w1270:i32, "error out"=w1269:errorcluster)  [unwired: 5 in]
                        n598 = call "AMC_controlRtOutSignalMode.vi"("deviceHandle"=w1271, "mode in"=w1270, "error in"=w1269, "set"=FALSE) -> ("mode out"=w1266:i32, "error out"=w1268:errorcluster)  [unwired: 4 in, 1 out]
                        n599 = local write "Output Mode"(w1266) -> ()
                      }
                      event "AquadB out 3": Value Change {
                        n600 = event-data() -> ()  [unwired: 1 in, 1 out]
                        n601 = call "AMC_controlAQuadBOut.vi"("set"=TRUE, "enable in"="AquadB out 3", "axis"=w1284, "deviceHandle"=w1283) -> ("error out"=w1278:errorcluster, "axis"=w1279:u8, "deviceHandle"=w1280:i32)  [unwired: 4 in, 1 out]
                        n602 = call "AMC_controlAQuadBOut.vi"("set"=FALSE, "error in"=w1278, "axis"=w1279, "deviceHandle"=w1280) -> ("error out"=w1277:errorcluster, "enable out"=w1275:bool)  [unwired: 4 in, 2 out]
                        n603 = local write "AquadB out 3"(w1275) -> ()
                      }
                      event "AqaudB clock 3": Value Change {
                        n604 = event-data() -> ()  [unwired: 1 in, 1 out]
                        n605 = call "AMC_controlAQuadBOutClock.vi"("set"=TRUE, "clock in"="AqaudB clock 3", "axis"=w1291, "deviceHandle"=w1292) -> ("error out"=w1287:errorcluster, "axis"=w1288:u8, "deviceHandle"=w1289:i32)  [unwired: 4 in, 1 out]
                        n606 = call "AMC_controlAQuadBOutClock.vi"("set"=FALSE, "error in"=w1287, "axis"=w1288, "deviceHandle"=w1289) -> ("error out"=w1286:errorcluster, "clock out"=w1285:i32)  [unwired: 4 in, 2 out]
                        n607 = local write "AqaudB clock 3"(w1285) -> ()
                      }
                      event "AquadB Resolution 3": Value Change {
                        n608 = event-data() -> ()  [unwired: 1 in, 1 out]
                        n609 = call "AMC_controlAQuadBOutResolution.vi"("set"=TRUE, "resolution in"="AquadB Resolution 3", "axis"=w1301, "deviceHandle"=w1302) -> ("error out"=w1299:errorcluster, "axis"=w1297:u8, "deviceHandle"=w1298:i32)  [unwired: 4 in, 1 out]
                        n610 = call "AMC_controlAQuadBOutResolution.vi"("set"=TRUE, "error in"=w1299, "axis"=w1297, "deviceHandle"=w1298) -> ("error out"=w1296:errorcluster, "resolution out"=w1295:i32)  [unwired: 4 in, 2 out]
                        n611 = local write "AquadB Resolution 3"(w1295) -> ()
                      }
                      event "Reset Error 6": Value Change {
                        n612 = event-data() -> ()  [unwired: 1 in, 1 out]
                        n613 = local write "Error 6"(FALSE ("Error 6")) -> ()
                        n614 = local write "Error Message 6"("" ("Error Message")) -> ()
                      }
                    }
                    n615 = Unbundle(w1174) -> ("code"=w1176:i32, "source"=w1177:string)  [unwired: 1 out]
                    n616 = Not Equal To 0?(x=w1176) -> (x != 0?=w1175:bool)
                    n617 = case shown="True" w1175 {
                      selector: w1175 -> [_ w1181]
                      tunnel: w1177 -> [_ w1182]
                      frame False {
                      }
                      frame True {
                        "Error Message 6" <- w1182
                        "Error 6" <- w1181
                      }
                    }
                  }
                }
              }
              frame "About" {
                n618 = event shown="[3] \"Unlock\": Value Change" {
                  selector: _ -> [_ _ _ _ _ _ _ _]
                  dyn-events: _ -> [_ _ _ _ _ _ _ _]
                  timeout: 1 -> [_ _ _ _ _ _ _ _]
                  tunnel: w1311 -> [w1321 w1323 w1326 w1329 w1331 w1334 w1336 _]
                  tunnel: [w1316 w1322 w1325 w1328 w1330 w1333 w1335 _] -> w1307
                  event Timeout {
                    n619 = event-data() -> ()  [unwired: 1 in, 1 out]
                    n620 = call "AMC_getLockStatus.vi"("deviceHandle"=w1321) -> ("error out"=w1317:errorcluster, "locked"=→"locked":bool, "authorized"=→"authorized":bool, "deviceHandle"=w1318:i32)  [unwired: 7 in]
                    n621 = call "AMC_getDeviceName.vi"("error in"=w1317, "deviceHandle"=w1318) -> ("error out"=w1316:errorcluster, "name"=→"Name":string)  [unwired: 7 in, 1 out]
                  }
                  event "name": Value Change {
                    n622 = event-data() -> ()  [unwired: 1 in, 1 out]
                    n623 = call "AMC_setDeviceName.vi"("name"="name", "deviceHandle"=w1323) -> ("error out"=w1322:errorcluster)  [unwired: 8 in, 1 out]
                  }
                  event "Lock password": Value Change {
                    n624 = event-data() -> ()  [unwired: 1 in, 1 out]
                    n625 = call "AMC_lock.vi"("password"="Lock password", "deviceHandle"=w1326) -> ("error out"=w1325:errorcluster)  [unwired: 8 in, 1 out]
                  }
                  event "Unlock": Value Change {
                    n626 = event-data() -> ()  [unwired: 1 in, 1 out]
                    n627 = call "AMC_unlock.vi"("deviceHandle"=w1329) -> ("error out"=w1328:errorcluster)  [unwired: 9 in, 1 out]
                  }
                  event "Access Password": Value Change {
                    n628 = event-data() -> ()  [unwired: 1 in, 1 out]
                    n629 = call "AMC_grantAccess.vi"("password"="Access Password", "deviceHandle"=w1331) -> ("error out"=w1330:errorcluster)  [unwired: 8 in, 1 out]
                  }
                  event "Reboot": Value Change {
                    n630 = event-data() -> ()  [unwired: 1 in, 1 out]
                    n631 = call "AMC_rebootSystem.vi"("deviceHandle"=w1334) -> ("error out"=w1333:errorcluster)  [unwired: 9 in, 1 out]
                  }
                  event "Factory Reset": Value Change {
                    n632 = event-data() -> ()  [unwired: 1 in, 1 out]
                    n633 = call "AMC_factoryReset.vi"("deviceHandle"=w1336) -> ("error out"=w1335:errorcluster)  [unwired: 9 in, 1 out]
                  }
                  event "Reset Error 7": Value Change {
                    n634 = event-data() -> ()  [unwired: 1 in, 1 out]
                    n635 = local write "Error 7"(FALSE ("Error 7")) -> ()
                    n636 = local write "Error Message 7"("" ("Error Message 9")) -> ()
                  }
                }
                n637 = Unbundle(w1307) -> ("code"=w1309:i32, "source"=w1310:string)  [unwired: 1 out]
                n638 = Not Equal To 0?(x=w1309) -> (x != 0?=w1308:bool)
                n639 = case shown="True" w1308 {
                  selector: w1308 -> [_ w1313]
                  tunnel: w1310 -> [_ w1314]
                  frame False {
                  }
                  frame True {
                    "Error Message 7" <- w1314
                    "Error 7" <- w1313
                  }
                }
              }
            }
          }
        }
        frame #2 {
          # "Disconnecting"
          n640 = call "AMC_close.vi"("deviceHandle"=w1339) -> ()  [unwired: 6 in, 1 out]
          n641 = local write "stop"(FALSE ("stop")) -> ()
        }
      }
    }
    frame True {
      # "No Devices Found"
      n642 = while {
        stop <- w1341 stop-if-true
        # "No Device Massage"
        n643 = One Button Dialog(message="No Devices Found", button name ("OK")="OK") -> (true=w1341:bool)
      }
    }
  }
